vi "ZVisualize.vi"() -> ()   [LabVIEW 2016]
uses:
  <vilib>/Utility/miscctls.llb/LVPointDoubleTypeDef.ctl
  subVI/ZDataVIS_StateWire.ctl
  <vilib>/MakerHub/Toolbox/LMH-Toolbox.lvlib
  <userlib>/_OpenG.lib/array/array.llb/Reverse 2D Array (DBL)__ogtk.vi
panel:
  out "mem after unflatten":dbl
  out "mem before unflatten":dbl
  out "mem after load dat":dbl
  out "mem before load dat":dbl
  out "after 'graph smoething'":dbl
  out "before 'graph something'":dbl
  out "Vfast":dbl[](graph)
  in  "scannn names":string[](array[string])
  in  "IV setup":T1={"# of Vslow"=1, "# Vfast"=41, "#IV Curves at each gate"=1, "B/T offset"=0, "Discard first # curves"=0, "Manual offset"=0, "Field Period"=1, "# of fields/Temperatures"=1}
  in  "Vsd":u16(ring)=17 items=["time", "temp", "B", "Vsource", "Lockin0", "Lockin1", "Lockin2", "Lockin3", "Lockin4", "Lockin5", "B_rate", "DC0", "DC1", "DC2", "DC3", "DC4", "DC5", "DC6", "DC7", "LOCKIN INFO"]
  in  "I":u16(ring)=5 items=["time", "temp", "B", "Vsource", "Lockin0", "Lockin1", "Lockin2", "Lockin3", "Lockin4", "Lockin5", "B_rate", "DC0", "DC1", "DC2", "DC3", "DC4", "DC5", "DC6", "DC7", "LOCKIN INFO"]
  out "wiring":string[][](array[string])
  in  "loading":bool=TRUE
  in  "Tab Control":T2(tab)
  in  "Z Axis":T3(ring)=enum."dI/dV 2T"
  in  "Y AXIS":i32(listbox)=7
  in  "X AXIS":i32(listbox)=1
  in  "tpose":bool
  in  "-Z":bool
  in  "-X":bool
  in  "-Y":bool
  in  "-X rows or columns":enum16{"rows", "columns"}(ring)
  in  "color scale":u32[](array[colorbox])=[16711680, 16772608, 6618880, 3381759, 16860, 10420479]
  in  "autoName axes":bool=TRUE
  in  "auto chop IV":bool=TRUE
  in  "e^2/h?":bool
  in  "Filter data?":bool
  in  "Differential Bin":dbl=10.0
  in  "Fake Point Val":dbl format="%#_13g"
  in  "X Scale Selection":enum32{"Manual", "Auto"}(tab)=enum."Auto"
  in  "Manual CTLs":T4={"X Low"=-0.2, "X High"=0.2, "X Step Size"=0.0005} {"X Step Size" format="%#_6p"; "X High" format="%#_6p"; "X Low" format="%#_6p"}
  in  "Auto CTLs":cluster{"METHOD":bool, "Steps":dbl}={"METHOD"=FALSE, "Steps"=1000.0}
  in  "Sweep Cursor":bool
  out "y direction":i32=1000
  out "x direction":i32=41
  in  "x or y sweep":enum32{"X", "Y"}(radio)
  in  "ms to wait":u32=5
  in  "loop ctl":bool
  in  "GENERATE BEFORE VISUALIZING":bool=TRUE
  in  "DAT GENERATION PARAMETERS":T5(tab)
  in  "File Information":T6={"File or folder path (input)"=path "G:/My Drive/ansom/Data/PPMS2/SA03008L.20190612/004_SG_IV_Testing", "output file description"="test123"}
  in  "increment (T) or overwrite (F) folders":bool
  in  "offset":i32
  in  "length":i32=100000
  in  "Portion of data":cluster{dbl, dbl}(slide)={1.0, 0.0} scale=0.0..1.0
  in  "attempt to fix filtered time?":bool
  in  "decimating factor for generation":i32=1
  out "Source-drain Current vs Voltage":cluster{"Vfast":dbl[], dbl[]}(graph) caption="XY Graph"
  out "Source-drain Current vs Side Gate Voltage":cluster{"Vfast":dbl[], dbl[]}(graph) caption="XY Graph"
  in  "update":bool
  out "Field":dbl=-5.021235521235521
  out "slowest":dbl=0.20001035419657615
  out "2term Intensity":dbl[][](graph)
  in  "side points 4T":i32=8
  in  "side points 2T":i32=12
  in  "Field/Temperature":i32(slide) min=0 max=36 step=1 scale=-1.1..-1.0
  out "Data Selection":cluster{dbl[], dbl[]}(graph)
  in  "OK":bool
  in  "USELESS CONTROLS":u32(colorbox)=6618880
  # "<- necessary if trying to nab"
  # "for 7/18/18"
  # "The Wayside™"
  # "for 6/__/19"
  # "**These switches don't\nupdate the axes yet"
  # "#TODO: add reverse feature"
  # "For old data -v"
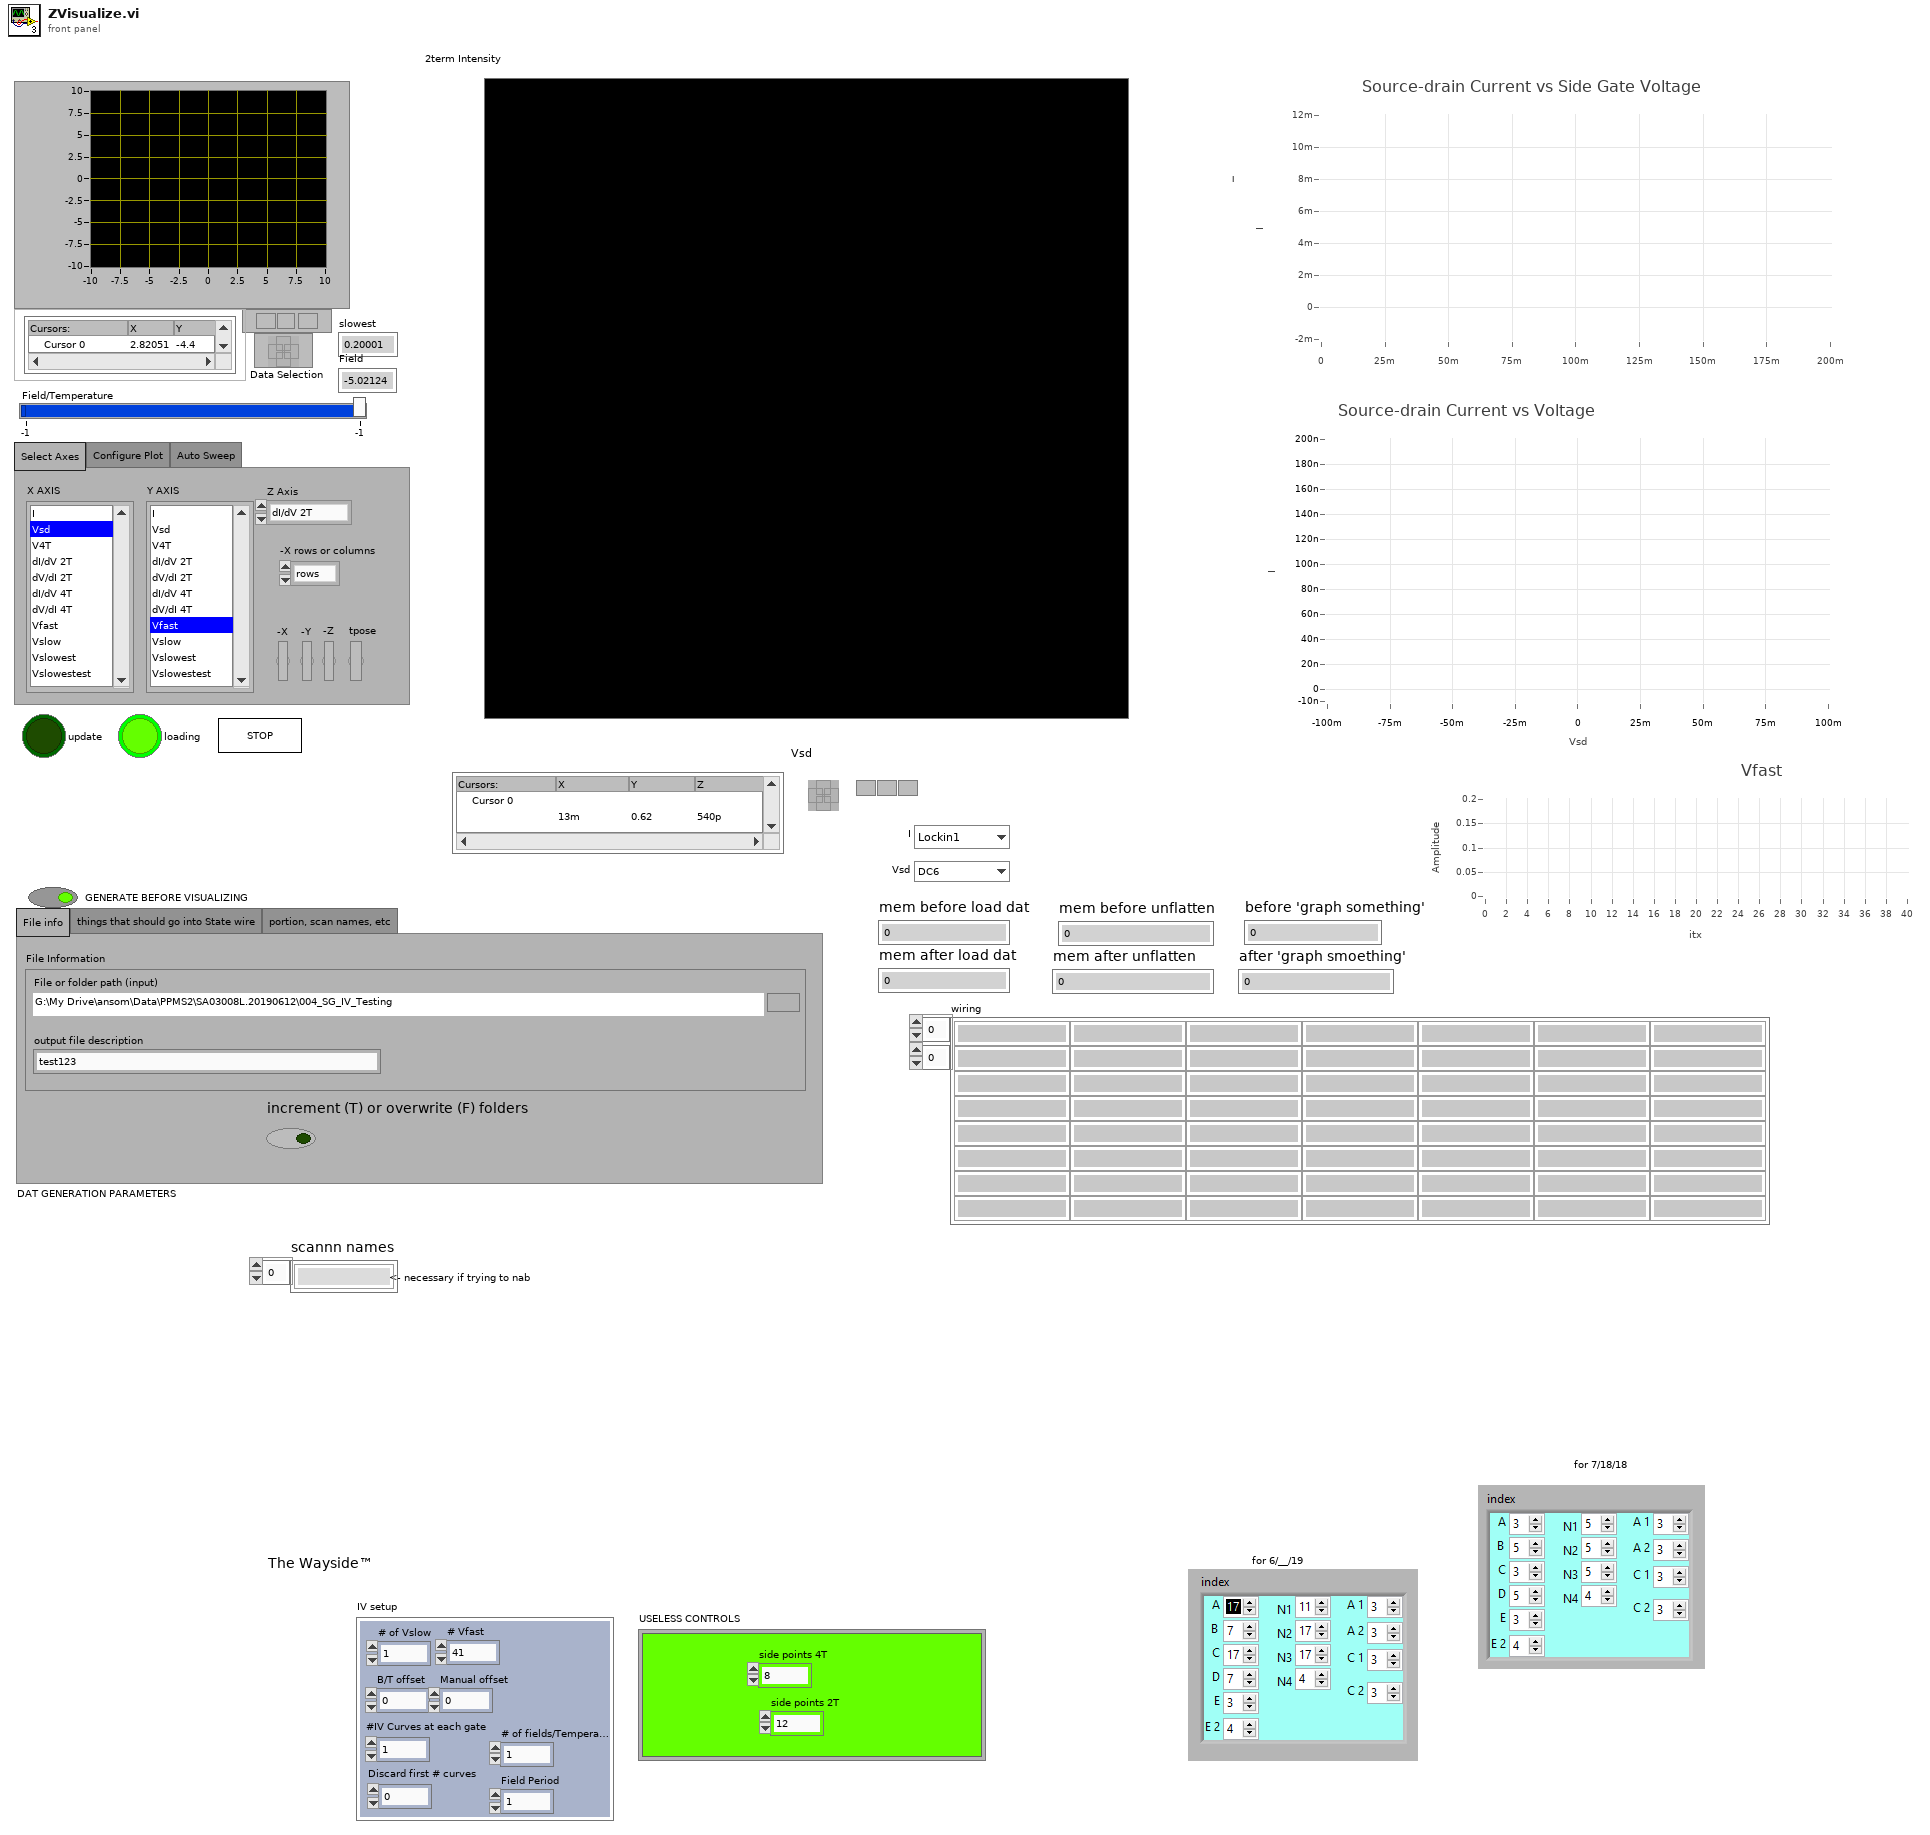
[diagram p1: front panel]
types:
  T1 = cluster{"# of Vslow":i32, "# Vfast":i32, "#IV Curves at each gate":i32, "B/T offset":i32, "Discard first # curves":i32, "Manual offset":i32, "Field Period":i32, "# of fields/Temperatures":i32}
  T2 = enum32{"Select Axes", "Configure Plot", "Auto Sweep"}
  T3 = enum16{"I", "Vsd", "V4T", "dI/dV 2T", "dV/dI 2T", "dV/dI 4T", "dI/dV 4T"}
  T4 = cluster{"X Low":dbl, "X High":dbl, "X Step Size":dbl}
  T5 = enum32{"File info", "things that should go into State wire", "portion, scan names, etc"}
  T6 = cluster{"File or folder path (input)":path, "output file description":string}
  T7 = enum32{"invalid app kind", "Development System", "Run Time System", "Student Edition", "Embedded LabVIEW", "Evaluation", "Custom"}
  T8 = cluster{"I":dbl[], "Vsd":dbl[], "V4T":dbl[], "dI/dV 2T":dbl[], "dV/dI 2T":dbl[], "dV/dI 4T":dbl[], "dI/dV 4T":dbl[]}[][][]
  T9 = enum32{"Invalid", "Standard", "Closed", "Hidden", "Minimized", "Maximized"}
  T10 = cluster{"# Vslow":i32, "# Vfast":i32, "# Vslowest":i32, "# Samples per IV":i32}
  T11 = typedef "ZDataVIS_StateWire.ctl" = cluster{"Core":cluster{"Current VI Reference":refnum<vi>, "Close Panel on Exit?":bool}, "Sweep Data Cluster":cluster{"Vfast":dbl[][], "Vslow":dbl[], "Vslowest":dbl[], "Comments":string, "Scan names":string[]}, "Cursor Info":cluster{"Fast Index":dbl[], "Slow Index":dbl, "Slow Indices":dbl[], "Raw Cursor Position":T12, "Field / temp":i32}, "Scan names":string[], "Data DVR":refnum<data-value>, "Arr of Y arrays (intensity info)":dbl[][], "Decimated X values":dbl[], "X Step Info":cluster{"X Low":dbl, "X High":dbl, "X Step":dbl}, "Voffset -2T":dbl, "Wiring Configuration ":string[][]}
  T12 = typedef "LVPointDoubleTypeDef.ctl" = cluster{"X":dbl, "Y":dbl}
  T13 = cluster{"Fast Index (Cursor X)":dbl[], "Slow Index (Cursor Y)":dbl, "Slow Indices":dbl[], "Raw Cursor Position":T12}
  T14 = cluster{"Vfast":dbl[][], "Vslow":dbl[], "Vslowest":dbl[], "Comments":string, "Scan names":string[]}
  T15 = cluster{"Current VI Reference":refnum<vi>, "Close Panel on Exit?":bool}
  T16 = typedef "Dictionary Object RefNum__ogtk.ctl" = refnum<k1>
  T17 = cluster{"IV":cluster{dbl[], dbl[]}[][][], "IV-2T":cluster{dbl[], dbl[]}[][][], "Vfast":dbl[][], "Vslow":dbl[], "Vslowest":dbl[], "Comments":string, "Scan names":string[]}[]
  T18 = cluster{"IV":cluster{dbl[], dbl[]}[][][], "IV-2T":cluster{dbl[], dbl[]}[][][], "Vfast":dbl[][], "Vslow":dbl[], "Vslowest":dbl[], "Comments":string, "Scan names":string[]}
  T19 = cluster{"Value":i32, "Value":i32, "Value":enum16{"I", "Vsd", "V4T", "dI/dV 2T", "dV/dI 2T", "dV/dI 4T", "dI/dV 4T"}}
  T20 = cluster{"Slow Index":dbl, "Field/Temperature":i32, dbl}
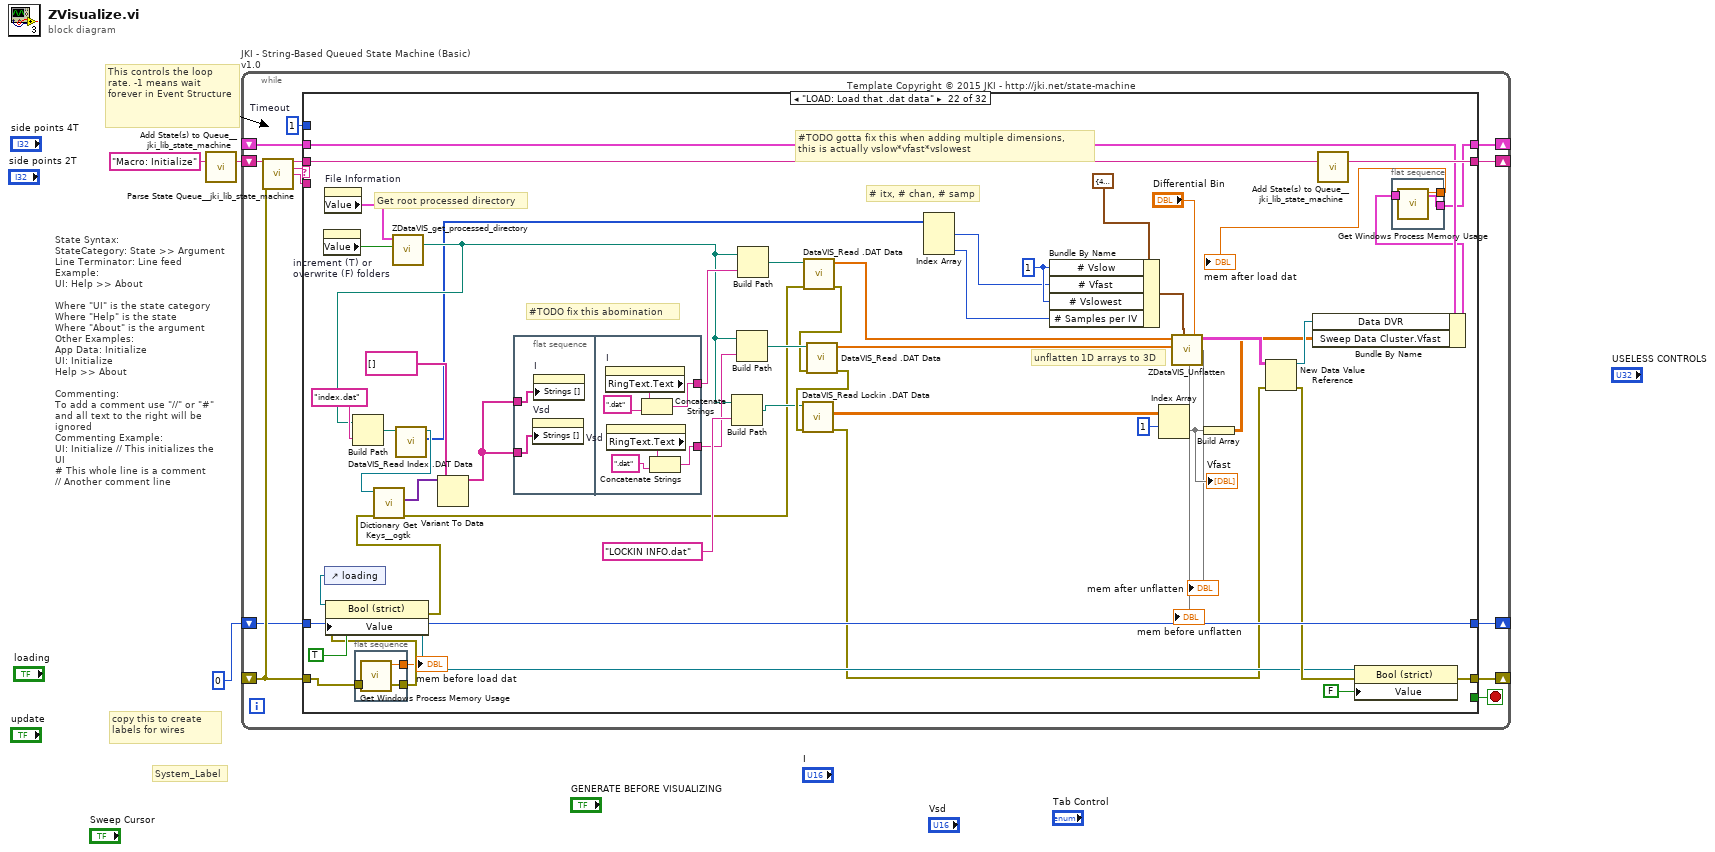
[diagram p0: block diagram]
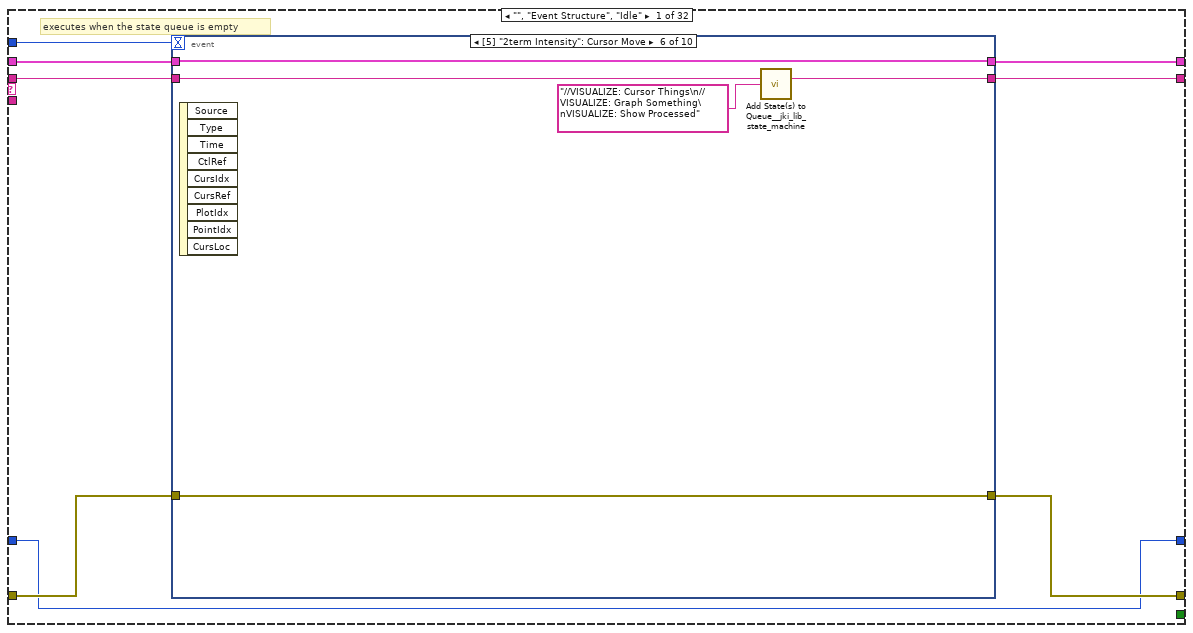
[diagram p2: hidden frame]
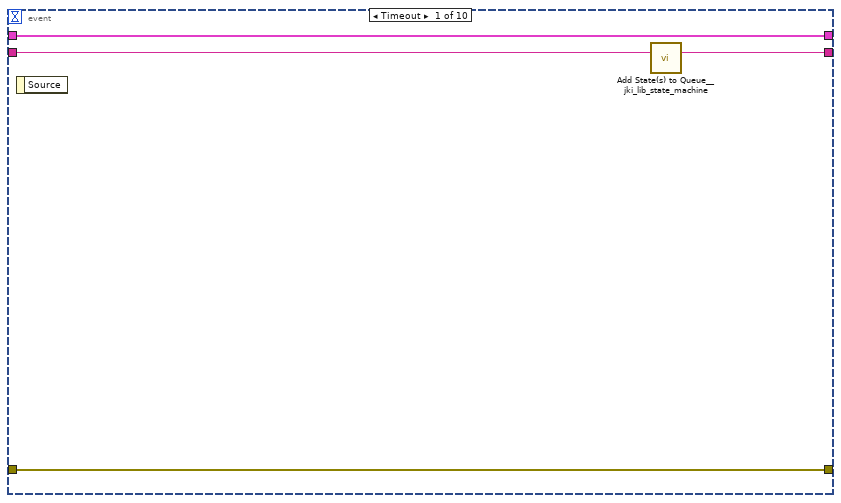
[diagram p3: hidden frame]
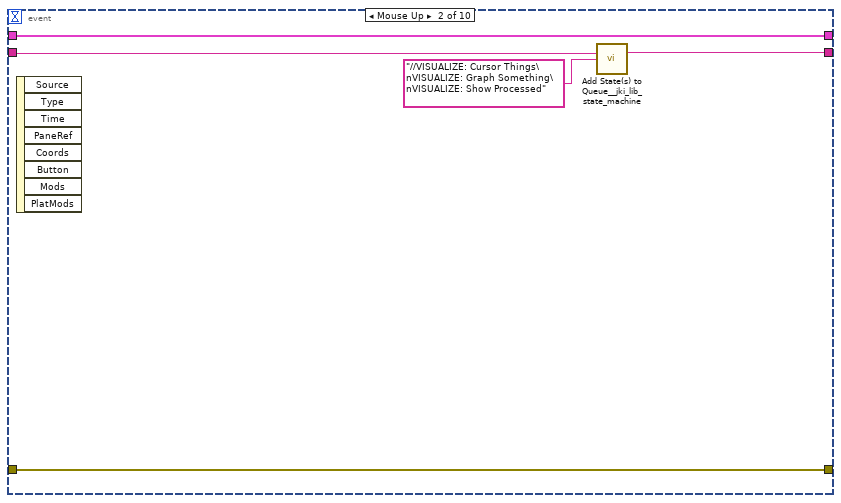
[diagram p4: hidden frame]
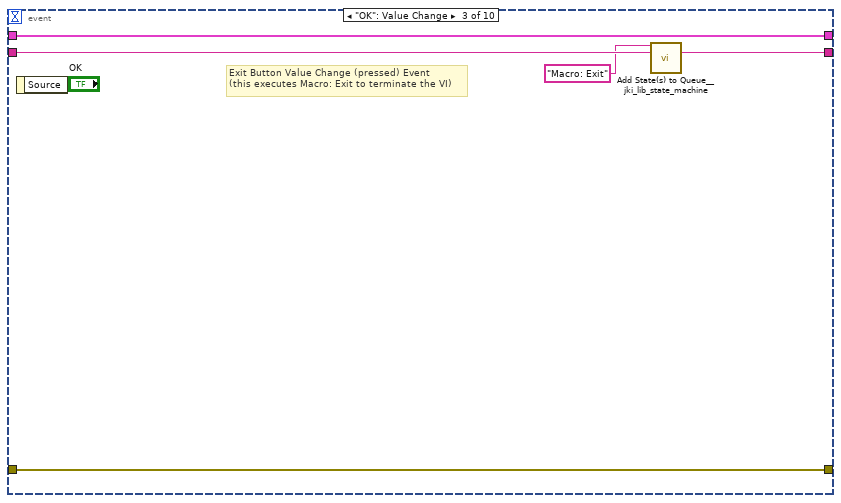
[diagram p5: hidden frame]
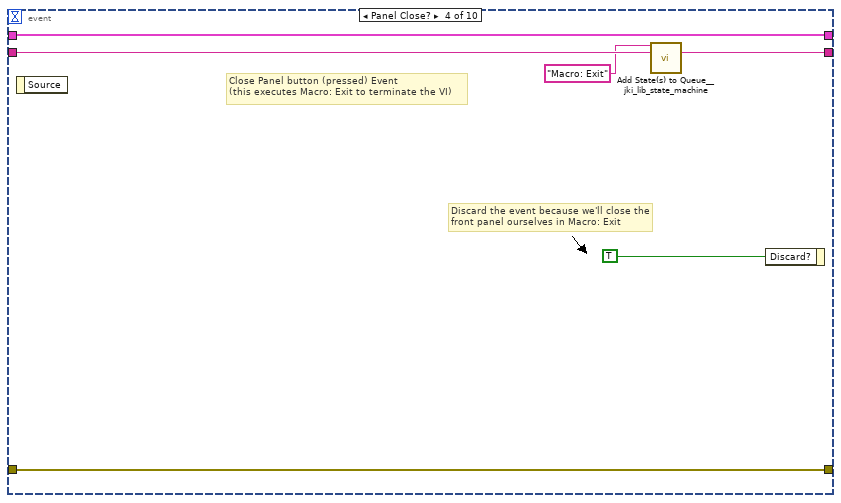
[diagram p6: hidden frame]
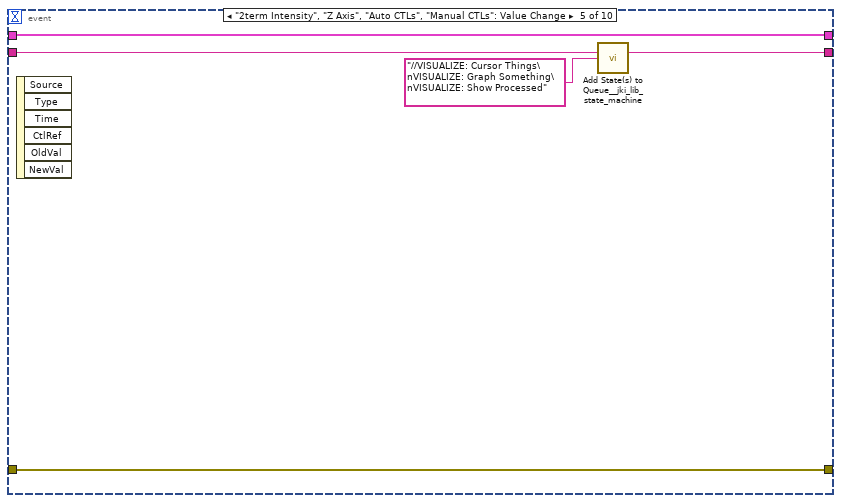
[diagram p7: hidden frame]
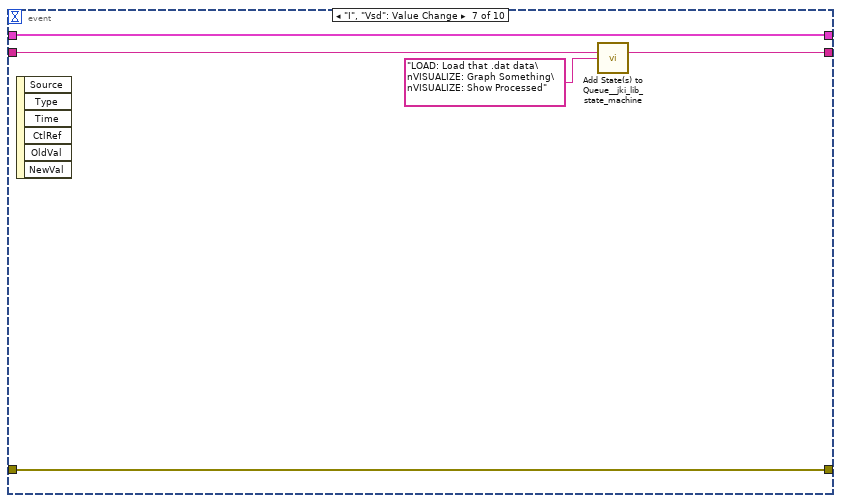
[diagram p8: hidden frame]
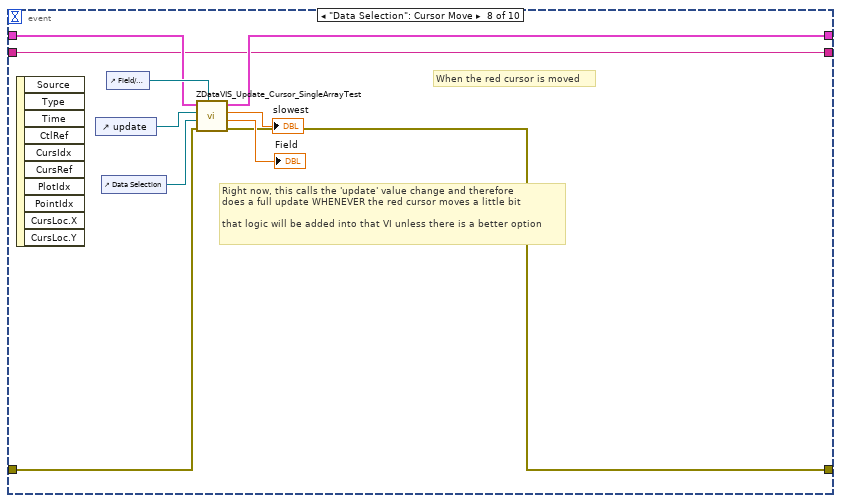
[diagram p9: hidden frame]
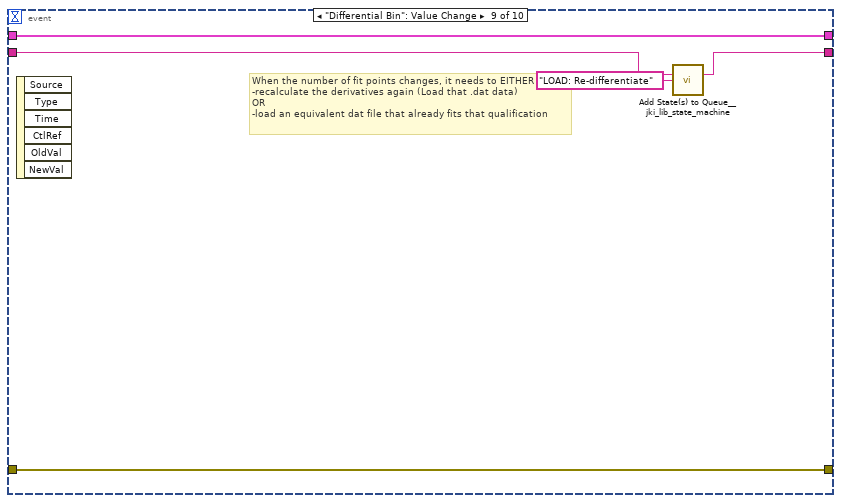
[diagram p10: hidden frame]
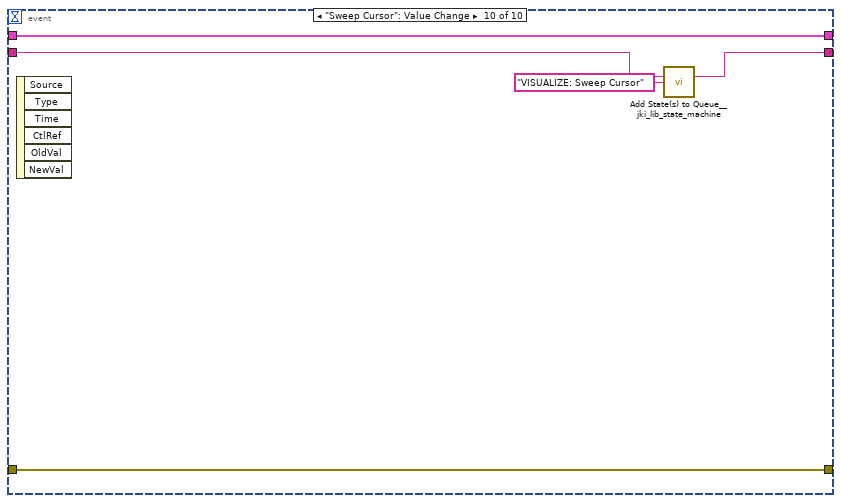
[diagram p11: hidden frame]
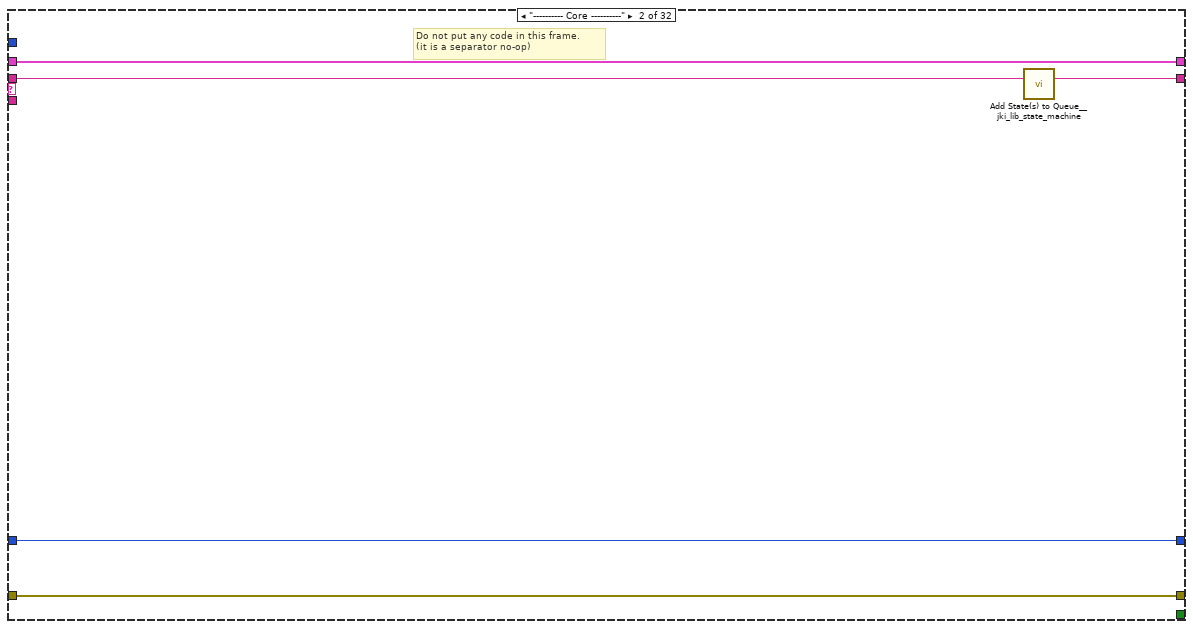
[diagram p12: hidden frame]
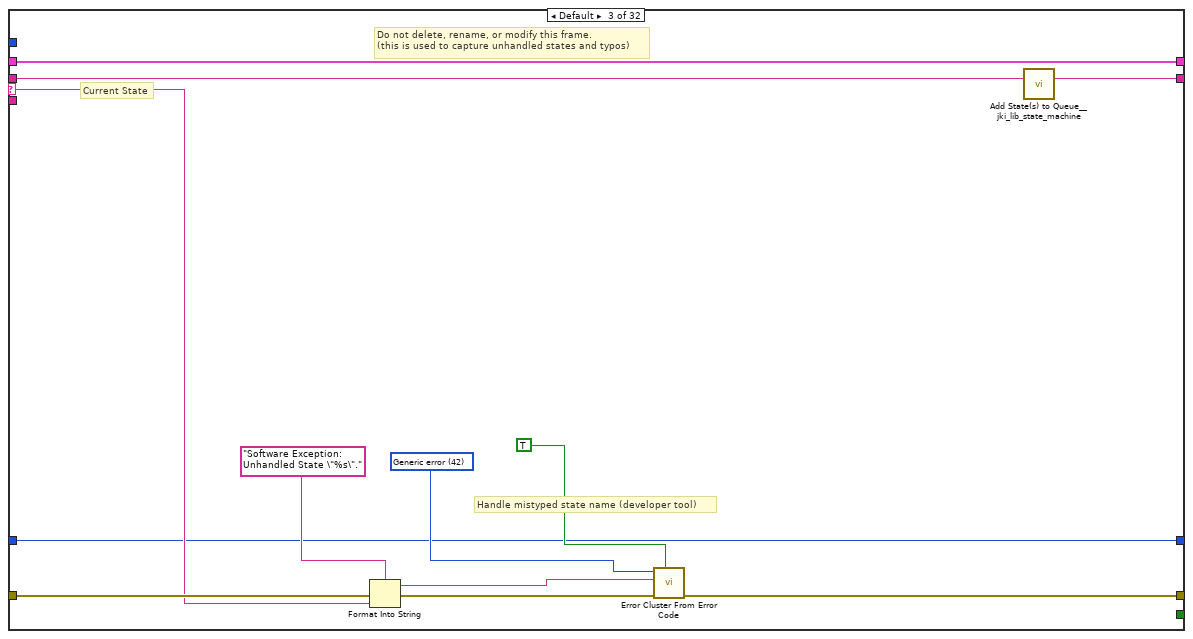
[diagram p13: hidden frame]
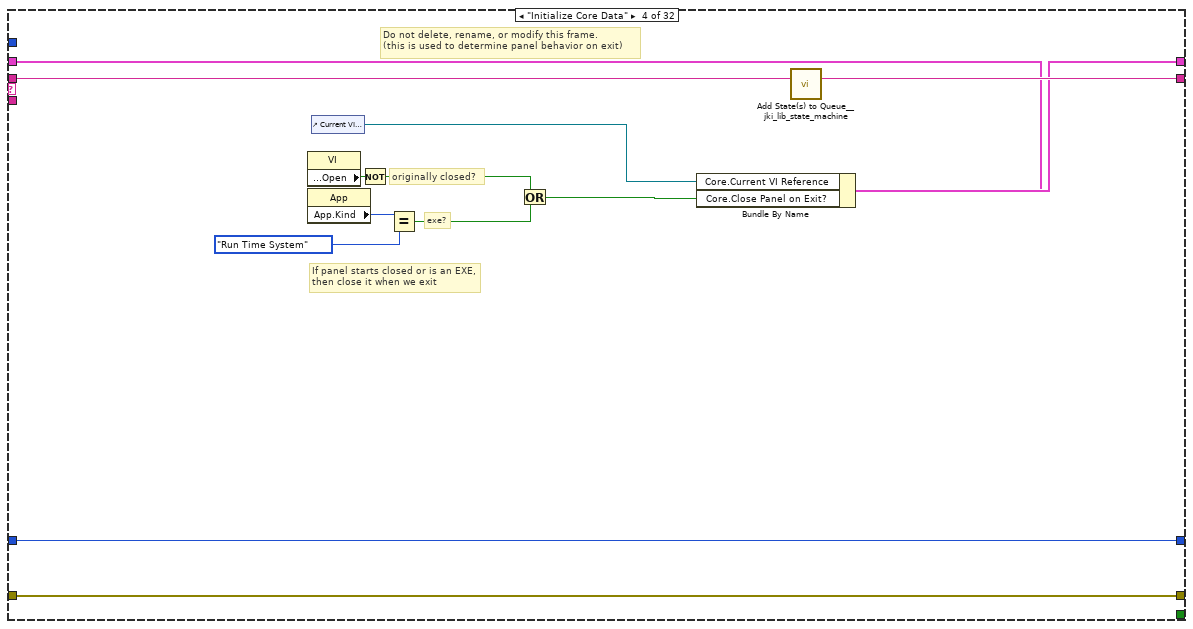
[diagram p14: hidden frame]
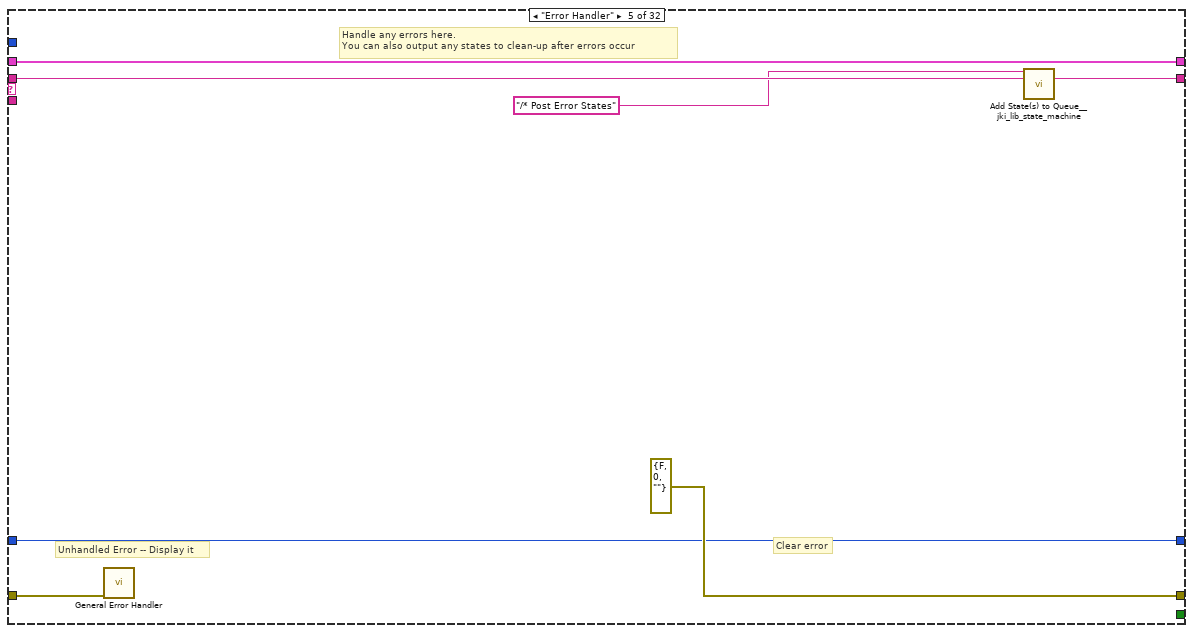
[diagram p15: hidden frame]
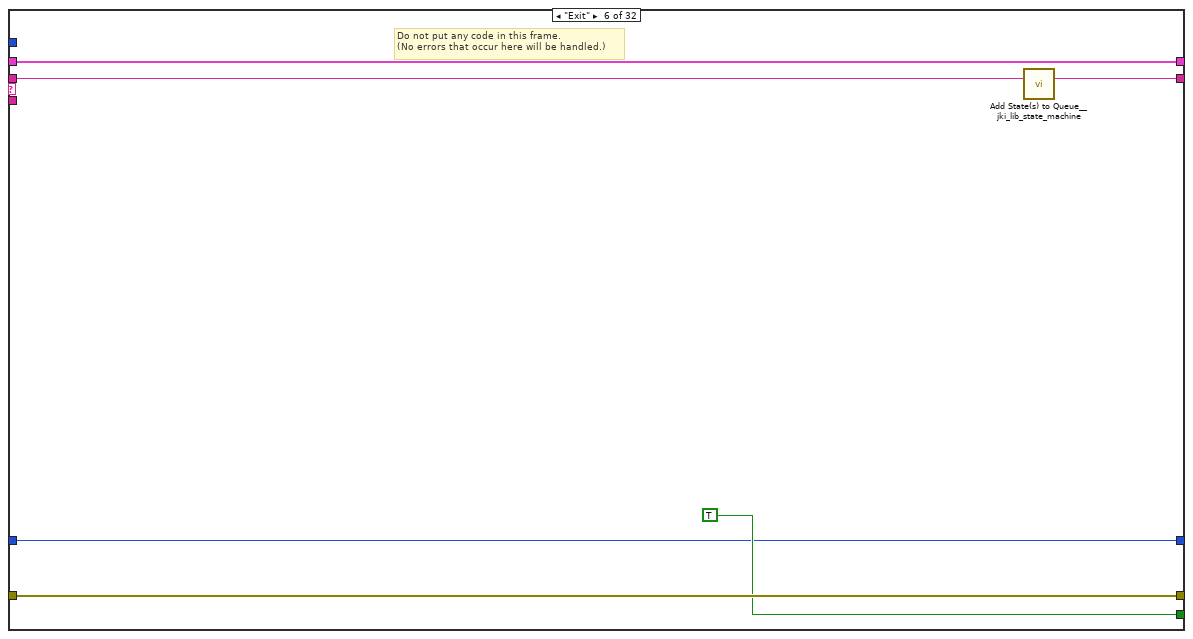
[diagram p16: hidden frame]
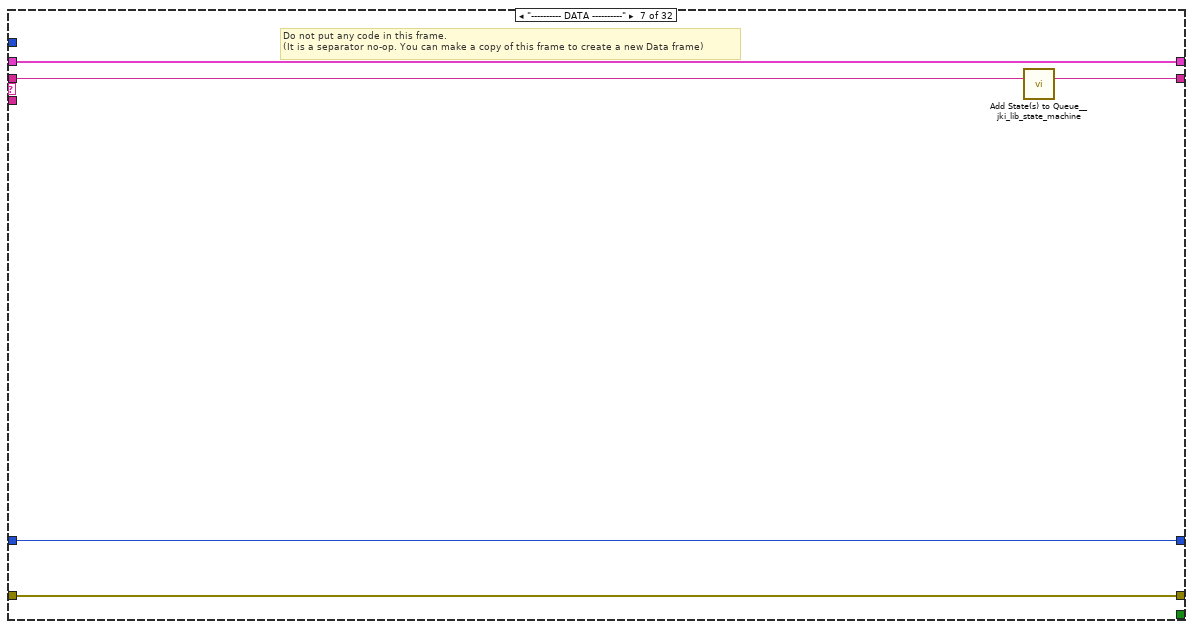
[diagram p17: hidden frame]
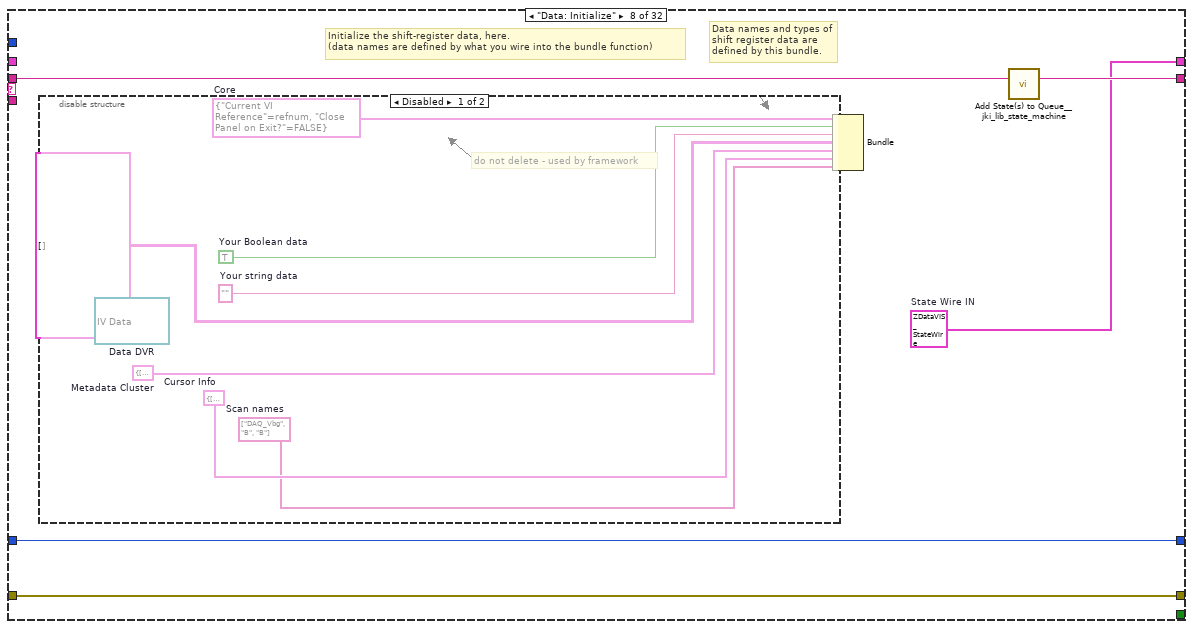
[diagram p18: hidden frame]
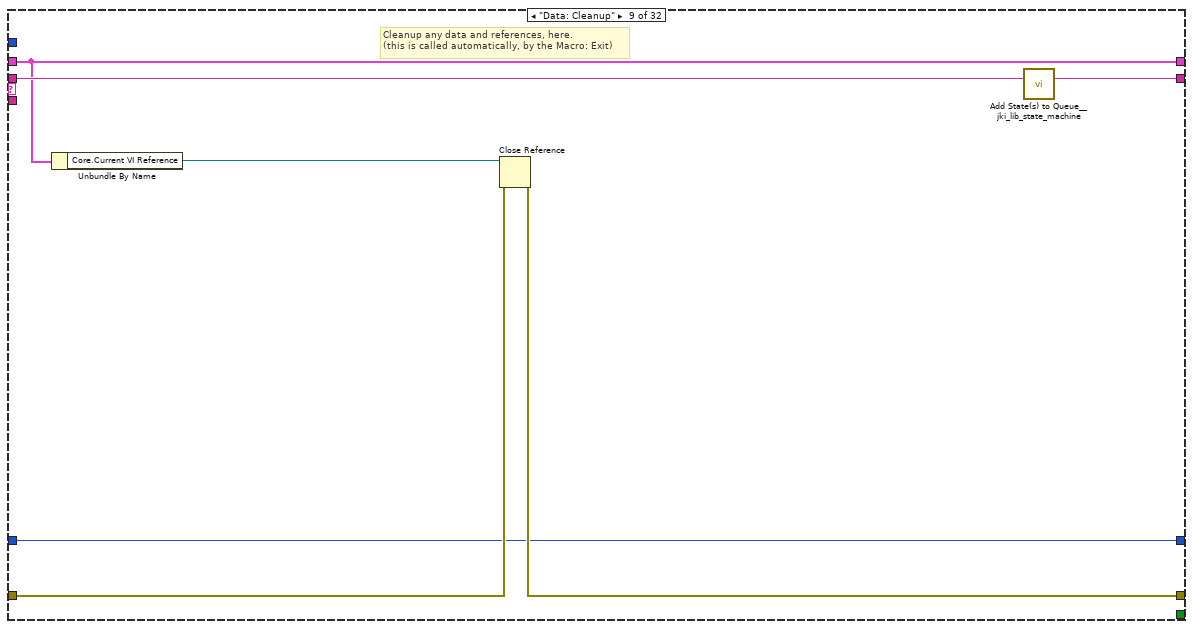
[diagram p20: hidden frame]
diagram:
  # "State Syntax:\nStateCategory: State >> Argument\nLine Terminator: Line feed\nExample:\nUI: Help >> About\n\nWhere \"UI\" is the state category\nWhere \"Help\" is the state\nWhere \"About\" is the argument\nOther Examples:\nApp Data: Initialize\nUI: Initialize\nHelp >> About\n\nCommenting:\nTo add a comment use \"//\" or \"#\" and all text to the right will be ignored\nCommenting Example:\nUI: Initialize // This initializes the UI\n# This whole line is a comment\n// Another comment line"
  # "copy this to create labels for wires"
  # "This controls the loop rate. -1 means wait forever in Event Structure"
  # "System_Label"
  n1 = call <vilib>:"Add State(s) to Queue__jki_lib_state_machine.vi"("State(s) in (\"\")"="Macro: Initialize") -> ("States Out"=w3:string)  [unwired: 14 in]
  n2 = while "JKI - String-Based Queued State Machine (Basic) v1.0" {
    shift-right: [w9] -> _
    shift-left: _ -> [w8]
    shift-right: [w12] -> _
    shift-left: _ -> [w6]
    shift-right: [w11] -> _
    shift-left: w3 -> [w13]
    shift-right: [w4] -> _
    shift-left: 0 -> [w5]
    stop <- w10 stop-if-true
    w7 = 1  # Timeout
    # "Template Copyright © 2015 JKI - http://jki.net/state-machine"
    n3 = call <vilib>:"Parse State Queue__jki_lib_state_machine.vi"("State Queue"=w13, "Error In (no error)"=w6) -> ("Remaining States"=w15:string, "Current State"=w16:string, "Arguments"=w14:string)  [unwired: 11 in]
    n4 = case shown="\"LOAD: Load that .dat data\"" w16 {
      selector: w16 -> [_ _ w86 _ _ _ _ _ _ _ _ _ _ _ _ _ _ _ _ _ _ _ _ _ _ _ _ _ _ _ _ _]
      tunnel: w15 -> [w24 w84 w90 w109 w116 w122 w127 w132 w146 w151 w156 w163 w175 w202 w208 w219 w231 w243 w248 w260 w265 w318 w358 w366 w396 w407 w434 w485 w499 w560 w568 w589]
      tunnel: w14 -> [_ _ _ _ _ _ _ _ _ _ _ w158 w169 _ _ _ _ _ _ _ _ _ _ _ _ _ _ _ _ _ _ _]
      tunnel: w8 -> [w22 w81 w88 w100 w113 w120 w124 _ w141 w148 w154 w161 w171 w199 w205 w216 w229 w240 w245 w258 w263 w316 w354 w362 w393 w404 w432 w469 w500 w557 w565 w587]
      tunnel: [w21 w82 w92 w106 errorcluster {"status"=FALSE, "code"=0, "source"=""} ("error out") w119 w125 w130 w142 w149 w153 w159 w172 w200 w206 w217 w226 w241 w246 w249 w262 w313 w336 w361 w385 w405 w417 w471 w501 w558 w566 w576] -> w12
      tunnel: w6 -> [w20 w82 w91 w106 w112 w119 w125 w130 w143 w149 w153 w160 w173 w200 w206 w217 w225 w241 w246 w256 w262 w273 w339 w361 w388 w405 w416 w472 w502 w558 w566 w577]
      tunnel: [w23 w83 w89 w108 w115 w121 w126 w131 w145 w150 w155 w162 w174 w201 w207 w218 w230 w242 w247 w259 w264 w317 w357 w365 w395 w406 w433 w484 w498 w559 w567 w588] -> w11
      tunnel: [_ _ _ _ _ TRUE _ _ _ _ _ _ _ _ _ _ _ _ _ _ _ _ _ _ _ _ _ _ _ _ _ _] -> w10
      tunnel: [w19 w81 w88 w107 w113 w120 w124 w129 w141 w148 w154 w161 w171 w199 w205 w216 w229 w240 w245 w258 w263 w269 w353 w364 w392 w404 w432 w468 w495 w557 w565 w587] -> w9
      tunnel: w7 -> [w18 _ _ _ _ _ _ _ _ _ _ _ _ _ _ _ _ _ _ _ _ _ _ _ _ _ _ _ _ _ _ _]
      tunnel: w5 -> [w17 w80 w85 w97 w110 w117 w123 w128 w140 w147 w152 w157 w168 w198 w203 w209 w228 w232 w244 w257 w261 w315 w340 w363 w390 w403 w423 w467 w493 w556 w561 w570]
      tunnel: [w17 w80 w85 w97 w110 w117 w123 w128 w140 w147 w152 w157 w168 w198 w203 w209 w228 w232 w244 w257 w261 w315 w340 w363 w390 w403 w426 w467 w493 w556 w561 w570] -> w4
      frame "", "Event Structure", "Idle" {
        # "executes when the state queue is empty"
        n5 = event shown="[5] \"2term Intensity\": Cursor Move" {
          selector: _ -> [_ _ _ _ _ _ _ _ _ _]
          dyn-events: _ -> [_ _ _ _ _ _ _ _ _ _]
          timeout: w18 -> [_ _ _ _ _ _ _ _ _ _]
          tunnel: w24 -> [w28 w32 w38 w44 w47 w52 w57 w64 w72 w76]
          tunnel: [w27 w30 w37 w43 w45 w50 w55 w64 w71 w75] -> w23
          tunnel: w22 -> [w25 w31 w35 w41 w49 w54 w59 w66 w73 w78]
          tunnel: [w26 w29 w36 w42 w48 w53 w58 w61 w74 w79] -> w21
          tunnel: w20 -> [w26 w29 w36 w42 w48 w53 w58 w63 w74 w79]
          tunnel: [w25 w31 w35 w41 w49 w54 w59 w65 w73 w78] -> w19
          event Timeout {
            n6 = event-data() -> ()  [unwired: 1 in, 1 out]
            n7 = call <vilib>:"Add State(s) to Queue__jki_lib_state_machine.vi"("State(s) in (\"\")"=w28) -> ("States Out"=w27:string)  [unwired: 14 in]
          }
          event Mouse Up {
            n8 = event-data() -> ()  [unwired: 1 in, 8 out]
            n9 = call <vilib>:"Add State(s) to Queue__jki_lib_state_machine.vi"("State(s) in (\"\")"=w32, "State(s) at Back (\"\")"="//VISUALIZE: Cursor Things\nVISUALIZE: Graph Something\nVISUALIZE: Show Processed" ("State(s) at Back (\"\")")) -> ("States Out"=w30:string)  [unwired: 13 in]
          }
          event "OK": Value Change {
            # "Exit Button Value Change (pressed) Event\n(this executes Macro: Exit to terminate the VI)"
            n10 = event-data() -> ()  [unwired: 1 in, 1 out]
            n11 = call <vilib>:"Add State(s) to Queue__jki_lib_state_machine.vi"("State(s) in Front (\"\")"="Macro: Exit", "State(s) in (\"\")"=w38) -> ("States Out"=w37:string)  [unwired: 13 in]
          }
          event Panel Close? {
            # "Discard the event because we'll close the front panel ourselves in Macro: Exit"
            # "Close Panel button (pressed) Event\n(this executes Macro: Exit to terminate the VI)"
            n12 = event-data() -> ()  [unwired: 1 in, 1 out]
            n13 = call <vilib>:"Add State(s) to Queue__jki_lib_state_machine.vi"("State(s) in Front (\"\")"="Macro: Exit", "State(s) in (\"\")"=w44) -> ("States Out"=w43:string)  [unwired: 13 in]
            n14 = event-data("Discard?"=TRUE) -> ()  [unwired: 1 in, 1 out]
          }
          event "2term Intensity", "Z Axis", "Auto CTLs", "Manual CTLs": Value Change {
            n15 = event-data() -> ()  [unwired: 1 in, 6 out]
            n16 = call <vilib>:"Add State(s) to Queue__jki_lib_state_machine.vi"("State(s) in (\"\")"=w47, "State(s) at Back (\"\")"="//VISUALIZE: Cursor Things\nVISUALIZE: Graph Something\nVISUALIZE: Show Processed" ("State(s) at Back (\"\")")) -> ("States Out"=w45:string)  [unwired: 13 in]
          }
          event "2term Intensity": Cursor Move {
            n17 = event-data() -> ()  [unwired: 1 in, 9 out]
            n18 = call <vilib>:"Add State(s) to Queue__jki_lib_state_machine.vi"("State(s) in (\"\")"=w52, "State(s) at Back (\"\")"="//VISUALIZE: Cursor Things\n//VISUALIZE: Graph Something\nVISUALIZE: Show Processed" ("State(s) at Back (\"\")")) -> ("States Out"=w50:string)  [unwired: 13 in]
          }
          event "I", "Vsd": Value Change {
            n19 = event-data() -> ()  [unwired: 1 in, 6 out]
            n20 = call <vilib>:"Add State(s) to Queue__jki_lib_state_machine.vi"("State(s) in (\"\")"=w57, "State(s) at Back (\"\")"="LOAD: Load that .dat data\nVISUALIZE: Graph Something\nVISUALIZE: Show Processed" ("State(s) at Back (\"\")")) -> ("States Out"=w55:string)  [unwired: 13 in]
          }
          event "Data Selection": Cursor Move {
            # "Right now, this calls the 'update' value change and therefore \ndoes a full update WHENEVER the red cursor moves a little bit\n\nthat logic will be added into that VI unless there is a better option"
            # "When the red cursor is moved"
            n21 = event-data() -> ()  [unwired: 1 in, 10 out]
            n22 = control-ref of="update"() -> (w62:refnum<vi>)
            n23 = control-ref of="Data Selection"() -> (w68:refnum<vi>)
            n24 = control-ref of="Field/Temperature"() -> (w67:refnum<vi>)
            n25 = call "ZDataVIS_Update_Cursor_SingleArrayTest.vi"("Field/Temperature 2"=w67, "error in (no error)"=w63, "Cursor Graph"=w68, "update bool"=w62, "State Wire IN 2"=w66) -> ("error out"=w61:errorcluster, "Field"=→"Field":dbl, "slowest"=→"slowest":dbl, "State Wire IN 3"=w65:T11)  [unwired: 3 in]
          }
          event "Differential Bin": Value Change {
            # "When the number of fit points changes, it needs to EITHER\n-recalculate the derivatives again (Load that .dat data)\nOR\n-load an equivalent dat file that already fits that qualification"
            n26 = event-data() -> ()  [unwired: 1 in, 6 out]
            n27 = call <vilib>:"Add State(s) to Queue__jki_lib_state_machine.vi"("State(s) in (\"\")"=w72, "State(s) at Back (\"\")"="LOAD: Re-differentiate" ("State(s) at Back (\"\")")) -> ("States Out"=w71:string)  [unwired: 13 in]
          }
          event "Sweep Cursor": Value Change {
            n28 = event-data() -> ()  [unwired: 1 in, 6 out]
            n29 = call <vilib>:"Add State(s) to Queue__jki_lib_state_machine.vi"("State(s) in (\"\")"=w76, "State(s) at Back (\"\")"="VISUALIZE: Sweep Cursor" ("State(s) at Back (\"\")")) -> ("States Out"=w75:string)  [unwired: 13 in]
          }
        }
      }
      frame "---------- Core ----------" {
        # "Do not put any code in this frame.\n(it is a separator no-op)"
        n30 = call <vilib>:"Add State(s) to Queue__jki_lib_state_machine.vi"("State(s) in (\"\")"=w84) -> ("States Out"=w83:string)  [unwired: 14 in]
      }
      frame Default {
        w95 = 42 items=["No error", "Argument error", "Memory is full", "Out of zone", "End of file", "File already open", "Generic file I/O error", "File not found", "File permission error", "Disk is full", "Duplicate path", "Too many files open", "System feature not enabled", "Resource file not found", "Cannot add resource", "Resource not found", "Image not found", "Image memory error", "Pen does not exist", "Config type invalid", "Config token not found", "Config parse error", "Config memory error", "Bad external code format", "Bad external code offset", "External code not present", "Null window", "Destroy window error", "Null menu", "Print aborted", "Bad print record", "Print driver error", "Windows error during printing", "Memory error during printing", "Print dialog error", "Generic print error", "Invalid device refnum", "Device not found", "Device parameter error", "Device unit error", "Cannot open device", "Device call aborted", "Generic error", "Cancelled by user", "Object ID too low", "Object ID too high", "Object not in heap", "Unknown heap", "Unknown object (invalid DefProc)", "Unknown object (DefProc not in table)", "Message out of range", "Invalid (null) method", "Unknown message", "Manager call not supported", "Bad address", "Network operation in progress", "Network operation timed out", "Connection is busy", "Network attribute not supported", "Network error", "Address in use", "System out of memory", "Connection aborted", "Connection refused", "Not connected", "Already connected", "Connection closed", "Initialization error (interapplication manager)", "Bad occurrence", "Wait on unbound occurrence handler", "Occurrence queue overflow", "Datalog type conflict", "Unused", "Unrecognized type (interapplication manager)", "Memory corrupt", "Failed to make temporary DLL", "Old CIN version", "Drag socket not found", "Failed to load drop-object", "Failed to register OLE object", "Failed to release OLE object", "Format specifier type mismatch", "Unknown format specifier", "Too few format specifiers", "Too many format specifiers", "Scan failed", "Newer CIN version", "Error converting to variant", "Runtime menu error", "Password tampered", "Variant attribute not found", "Incompatible variant data type", "Event data is not available", "Event Store is not present", "Occurrence is not found", "Event Queue is not created", "Event info is not available", "Refnum passed is NULL", "Error retrieving Class GUID", "Error retrieving CoClass GUID", "Error retrieving TypeLib GUID.", "Bad built application magic bytes.", "Specific driver is different from the specific driver associated with the Logical Name.", "There is no session opened to the class driver.", "Max Error", "MAX - Error with config objects", "MAX - Error loading configuration", "MAX - Group not supported"]
        # "Current State"
        # "Do not delete, rename, or modify this frame.\n(this is used to capture unhandled states and typos)"
        # "Handle mistyped state name (developer tool)"
        n31 = Format Into String(format string="Software Exception: Unhandled State \"%s\"." ("message"), error in=w91, w86) -> (resulting string=w94:string, error out=w93:errorcluster)  [unwired: 1 in]
        n32 = call <vilib>:"Error Cluster From Error Code.vi"("show call chain? (False)"=TRUE, "error in (no error)"=w93, "error message (\"\")"=w94, "error code (0)"=w95) -> ("error out"=w92:errorcluster)  [unwired: 5 in]
        n33 = call <vilib>:"Add State(s) to Queue__jki_lib_state_machine.vi"("State(s) in (\"\")"=w90) -> ("States Out"=w89:string)  [unwired: 14 in]
      }
      frame "Initialize Core Data" {
        # "Do not delete, rename, or modify this frame.\n(this is used to determine panel behavior on exit)"
        # "originally closed?"
        # "exe?"
        # "If panel starts closed or is an EXE, then close it when we exit"
        n34 = property class="VI"() -> ("Front Panel.Open"=w105:bool)  [unwired: 2 in, 2 out]
        n35 = property class="App"() -> ("App.Kind"=w104:T7)  [unwired: 2 in, 2 out]
        n36 = control-ref of="Current VI Reference"() -> (w98:refnum<vi>)
        n37 = Not(x=w105) -> (.not. x?=w102:bool)
        n38 = Equal?(x=w104, y=T7."Run Time System" ("Application:Kind")) -> (x = y?=w101:bool)
        n39 = Or(x=w102, y=w101) -> (x .or. y?=w99:bool)
        n40 = Bundle By Name(cluster=w100, "Core.Current VI Reference"=w98, "Core.Close Panel on Exit?"=w99) -> (w107:T11)
        n41 = call <vilib>:"Add State(s) to Queue__jki_lib_state_machine.vi"("State(s) in (\"\")"=w109) -> ("States Out"=w108:string)  [unwired: 14 in]
      }
      frame "Error Handler" {
        # "Unhandled Error -- Display it"
        # "Handle any errors here.\nYou can also output any states to clean-up after errors occur"
        # "Clear error"
        n42 = call <vilib>:"General Error Handler.vi"("error in (no error)"=w112) -> ()  [unwired: 10 in, 5 out]
        n43 = call <vilib>:"Add State(s) to Queue__jki_lib_state_machine.vi"("State(s) in Front (\"\")"="/* Post Error States", "State(s) in (\"\")"=w116) -> ("States Out"=w115:string)  [unwired: 13 in]
      }
      frame "Exit" {
        # "Do not put any code in this frame.\n(No errors that occur here will be handled.)"
        n44 = call <vilib>:"Add State(s) to Queue__jki_lib_state_machine.vi"("State(s) in (\"\")"=w122) -> ("States Out"=w121:string)  [unwired: 14 in]
      }
      frame "---------- DATA ----------" {
        # "Do not put any code in this frame.\n(It is a separator no-op. You can make a copy of this frame to create a new Data frame)"
        n45 = call <vilib>:"Add State(s) to Queue__jki_lib_state_machine.vi"("State(s) in (\"\")"=w127) -> ("States Out"=w126:string)  [unwired: 14 in]
      }
      frame "Data: Initialize" {
        w129 = T11 {"Core"={"Current VI Reference"=refnum, "Close Panel on Exit?"=FALSE}, "Sweep Data Cluster"={"Vfast"=[], "Vslow"=[], "Vslowest"=[], "Comments"="", "Scan names"=[]}, "Cursor Info"={"Fast Index"=[], "Slow Index"=0.0, "Slow Indices"=[], "Raw Cursor Position"={"X"=0.0, "Y"=0.0}, "Field / temp"=0}, "Scan names"=[], "Data DVR"=refnum, "Arr of Y arrays (intensity info)"=[], "Decimated X values"=[], "X Step Info"={"X Low"=-0.1, "X High"=0.1, "X Step"=4e-05}, "Voffset -2T"=0.0, "Wiring Configuration "=[]}  # State Wire IN
        # "Data names and types of shift register data are defined by this bundle."
        # "Initialize the shift-register data, here.\n(data names are defined by what you wire into the bundle function)"
        n46 = disable-structure shown="Disabled" {
          frame Disabled {
            w134 = string[] ["DAQ_Vbg", "B", "B"]  # Scan names
            w135 = T13 {"Fast Index (Cursor X)"=[], "Slow Index (Cursor Y)"=0.0, "Slow Indices"=[], "Raw Cursor Position"={"X"=0.0, "Y"=0.0}}  # Cursor Info
            w136 = T14 {"Vfast"=[], "Vslow"=[], "Vslowest"=[], "Comments"="", "Scan names"=[]}  # Metadata Cluster
            (unwired) refnum<data-value> refnum  # Data DVR
            w137 = T15 {"Current VI Reference"=refnum, "Close Panel on Exit?"=FALSE}  # Core
            w138 = ""  # Your string data
            w139 = TRUE  # Your Boolean data
            # "do not delete - used by framework"
            n47 = Bundle("Core"=w137, "Your Boolean data"=w139, "Your string data"=w138, "Data Cell"=T8 [], "Metadata Cluster"=w136, "Cursor Info"=w135, "Scan names"=w134) -> ()  [unwired: 1 in, 1 out]
          }
          frame Enabled {
          }
        }
        n48 = call <vilib>:"Add State(s) to Queue__jki_lib_state_machine.vi"("State(s) in (\"\")"=w132) -> ("States Out"=w131:string)  [unwired: 14 in]
      }
      frame "Data: Cleanup" {
        # "Cleanup any data and references, here.\n(this is called automatically, by the Macro: Exit)"
        n49 = Unbundle By Name(w141) -> ("Core.Current VI Reference"=w144:refnum<vi>)
        n50 = Close Reference(reference=w144, error in (no error)=w143) -> (error out=w142:errorcluster)
        n51 = call <vilib>:"Add State(s) to Queue__jki_lib_state_machine.vi"("State(s) in (\"\")"=w146) -> ("States Out"=w145:string)  [unwired: 14 in]
      }
      frame "---------- UI ----------" {
        # "Do not put any code in this frame.\n(It is a separator no-op. You can make a copy of this frame to create a new UI frame)"
        n52 = call <vilib>:"Add State(s) to Queue__jki_lib_state_machine.vi"("State(s) in (\"\")"=w151) -> ("States Out"=w150:string)  [unwired: 14 in]
      }
      frame "UI: Initialize" {
        # "Initialize the User Interface, here.\n(this is called automatically, by the Macro: Init)"
        n53 = call <vilib>:"Add State(s) to Queue__jki_lib_state_machine.vi"("State(s) in (\"\")"=w156) -> ("States Out"=w155:string)  [unwired: 14 in]
      }
      frame "UI: Cursor Set" {
        # "Argument"
        # "Set and Unset Cursor Busy.\n(Usage: \"UI: Cursor Set >> Busy|Idle\")"
        n54 = case shown="\"Idle\", Default" w158 {
          tunnel: w160 -> [w165 w167]
          tunnel: [w164 w166] -> w159
          frame "Idle", Default {
            n55 = call <vilib>:"Unset Busy.vi"("error in (no error)"=w165) -> ("error out"=w164:errorcluster)  [unwired: 10 in]
          }
          frame "Busy" {
            n56 = call <vilib>:"Set Busy.vi"("error in (no error)"=w167) -> ("error out"=w166:errorcluster)  [unwired: 9 in, 1 out]
          }
        }
        n57 = call <vilib>:"Add State(s) to Queue__jki_lib_state_machine.vi"("State(s) in (\"\")"=w163) -> ("States Out"=w162:string)  [unwired: 14 in]
      }
      frame "UI: Front Panel State" {
        # "Argument"
        # "Set Front Panel Open or Closed\n(Usage: \"UI: Front Panel State >> Open|Close\")"
        n58 = Unbundle By Name(w171) -> ("Core.Current VI Reference"=w170:refnum<vi>)
        n59 = case shown="\"Open\", Default" w169 {
          tunnel: w173 -> [w179 w192]
          tunnel: [w181 w193] -> w172
          tunnel: w170 -> [w180 w190]
          frame "Open", Default {
            n60 = property class="VI"(reference=w180, error in=w179) -> (reference out=w177:refnum<vi>, error out=w178:errorcluster, "Front Panel.Open"=w176:bool)
            n61 = case shown="True" w176 {
              tunnel: [w184 w187] -> w181
              tunnel: w178 -> [w183 w187]
              tunnel: w177 -> [w182 _]
              frame False {
                n62 = invoke class="VI" method="FP.Open"(reference=w182, error in=w183, "Activate"=TRUE, "State"=T9."Standard") -> (error out=w184:errorcluster)  [unwired: 1 in, 4 out]
              }
              frame True {
              }
            }
          }
          frame "Close" {
            n63 = property class="VI"(reference=w190, error in=w192) -> (reference out=w189:refnum<vi>, error out=w191:errorcluster, "Front Panel.Open"=w188:bool)
            n64 = case shown="True" w188 {
              tunnel: [w194 w197] -> w193
              tunnel: w191 -> [w194 w196]
              tunnel: w189 -> [_ w195]
              frame False {
              }
              frame True {
                n65 = invoke class="VI" method="FP.Close"(reference=w195, error in=w196) -> (error out=w197:errorcluster)  [unwired: 1 in, 2 out]
              }
            }
          }
        }
        n66 = call <vilib>:"Add State(s) to Queue__jki_lib_state_machine.vi"("State(s) in (\"\")"=w175) -> ("States Out"=w174:string)  [unwired: 14 in]
      }
      frame "---------- Macro ----------" {
        # "Do not put any code in this frame.\n(It is a separator no-op. You can make a copy of this frame to create a new Macro frame)"
        n67 = call <vilib>:"Add State(s) to Queue__jki_lib_state_machine.vi"("State(s) in (\"\")"=w202) -> ("States Out"=w201:string)  [unwired: 14 in]
      }
      frame "Macro: Initialize" {
        # "Initialization Macro\n(This is called once, when the VI starts)"
        n68 = call <vilib>:"Add State(s) to Queue__jki_lib_state_machine.vi"("State(s) in Front (\"\")"="Data: Initialize\nInitialize Core Data\nUI: Initialize\nUI: Front Panel State >> Open\nMacro: LOAD\nMacro: Visualize", "State(s) in (\"\")"=w208) -> ("States Out"=w207:string)  [unwired: 13 in]
      }
      frame "Macro: Exit" {
        # "Exit Macro\n(This is called once, when the VI exits)"
        n69 = Unbundle By Name(w216) -> ("Core.Close Panel on Exit?"=w215:bool)
        n70 = Select(t="UI: Front Panel State >> Close", s=w215, f="") -> (s? t:f=w212:string)
        n71 = call <vilib>:"Add State(s) to Queue__jki_lib_state_machine.vi"("State(s) in (\"\")"=w212, "State(s) at Back (\"\")"="Data: Cleanup\nExit") -> ("States Out"=w210:string)  [unwired: 13 in]
        n72 = call <vilib>:"Add State(s) to Queue__jki_lib_state_machine.vi"("State(s) in Front (\"\")"=w210, "State(s) in (\"\")"=w219) -> ("States Out"=w218:string)  [unwired: 13 in]
      }
      frame "Macro: LOAD" {
        # "Exit Macro\n(This is called once, when the VI exits)"
        n73 = property on="GENERATE BEFORE VISUALIZING" class="Bool (strict)"(error in=w225) -> (error out=w226:errorcluster, "Value"=w227:bool)  [unwired: 1 in, 1 out]
        n74 = Select(t="GENERATE: generate data\n", s=w227, f="") -> (s? t:f=w222:string)
        n75 = Concatenate Strings(w222, "LOAD: Load that .dat data\n//LOAD: Parse Comments" ("State(s) in Front (\"\")")) -> (w220:string)
        n76 = call <vilib>:"Add State(s) to Queue__jki_lib_state_machine.vi"("State(s) in Front (\"\")"=w220, "State(s) in (\"\")"=w231) -> ("States Out"=w230:string)  [unwired: 13 in]
      }
      frame "Macro: VISUALIZE" {
        # "#TODO: move loading to a speciial case"
        # "Skip or don't skip filtering step"
        # "Exit Macro\n(This is called once, when the VI exits)"
        n77 = Select(t="VISUALIZE: Apply SG Filter", s="Filter data?", f="") -> (s? t:f=w237:string)
        n78 = call <vilib>:"Add State(s) to Queue__jki_lib_state_machine.vi"("State(s) in Front (\"\")"="VISUALIZE: Initialize Cursor Graph\nVISUALIZE: Initialize Color Tables" ("State(s) in Front (\"\")"), "State(s) in (\"\")"=w237, "State(s) at Back (\"\")"="//VISUALIZE: Cursor Things\nVISUALIZE: Graph Something\nVISUALIZE: Show Processed" ("State(s) at Back (\"\")")) -> ("States Out"=w236:string)  [unwired: 12 in]
        n79 = call <vilib>:"Add State(s) to Queue__jki_lib_state_machine.vi"("State(s) in Front (\"\")"=w236, "State(s) in (\"\")"=w243) -> ("States Out"=w242:string)  [unwired: 13 in]
      }
      frame "---------- GENERATE ----------" {
        # "Template Separator\n(You can make a copy of, or modify, this frame)"
        n80 = call <vilib>:"Add State(s) to Queue__jki_lib_state_machine.vi"("State(s) in (\"\")"=w248) -> ("States Out"=w247:string)  [unwired: 14 in]
      }
      frame "GENERATE: generate data" {
        # "Template Separator\n(You can make a copy of, or modify, this frame)"
        n81 = call "ZGenerate.vi"("File Information"="File Information", "attempt to fix filtered time?"="attempt to fix filtered time?", "decimating factor for generation"="decimating factor for generation", "offset"="offset", "length"="length", "error in"=w256, "increment (T) or overwrite (F) folders"="increment (T) or overwrite (F) folders") -> ("error out"=w249:errorcluster)  [unwired: 6 in, 2 out]
        n82 = call <vilib>:"Add State(s) to Queue__jki_lib_state_machine.vi"("State(s) in (\"\")"=w260) -> ("States Out"=w259:string)  [unwired: 14 in]
      }
      frame "---------- LOAD ----------" {
        # "Template Separator\n(You can make a copy of, or modify, this frame)"
        n83 = call <vilib>:"Add State(s) to Queue__jki_lib_state_machine.vi"("State(s) in (\"\")"=w265) -> ("States Out"=w264:string)  [unwired: 14 in]
      }
      frame "LOAD: Load that .dat data" {
        w305 = 1
        # "# itx, # chan, # samp"
        # "#TODO fix this abomination"
        # "Get root processed directory"
        # "#TODO gotta fix this when adding multiple dimensions,\nthis is actually vslow*vfast*vslowest"
        # "unflatten 1D arrays to 3D"
        n84 = property on="increment (T) or overwrite (F) folders" class="Bool (strict)"() -> ("Value"=w297:bool)  [unwired: 2 in, 2 out]
        n85 = property on="File Information" class="Clust (strict)"() -> ("Value"=w295:T6)  [unwired: 2 in, 2 out]
        n86 = control-ref of="loading"() -> (w310:refnum<vi>)
        n87 = property class="Bool (strict)"(reference=w310, error in=w272, "Value"=TRUE) -> (reference out=w311:refnum<vi>, error out=w286:errorcluster)
        n88 = flat-sequence {
          tunnel: w273 -> [w322]
          tunnel: [w322] -> w272
          tunnel: [w321] -> w271
          frame #0 {
            n89 = call "Get Windows Process Memory Usage.vi"() -> ("Memory Used By This Process (KB)"=w321:dbl)  [unwired: 11 in]
          }
        }
        n90 = call "ZDataVIS_get_processed_directory.vi"("increment (T) or overwrite (F) folders"=w297, "File Information"=w295) -> ("modified path"=w280:path)  [unwired: 9 in]
        n91 = Build Path(base path=w280, name or relative path="index.dat") -> (appended path=w288:path)
        n92 = call "DataVIS_Read Index .DAT Data.vi"("file path (use dialog)"=w288) -> ("itx # info"=w276:i32[], "channel / path dictionary"=w284:T16)  [unwired: 8 in, 1 out]
        n93 = call <userlib>:"Dictionary Get Keys__ogtk.vi"("error in (no error)"=w286, "dictionary"=w284) -> ("error out"=w285:errorcluster, "keys"=w283:variant[])  [unwired: 7 in, 1 out]
        n94 = Variant To Data(type=string[] [], Variant=w283) -> (data=w278:string[])  [unwired: 1 in, 1 out]
        n95 = flat-sequence {
          tunnel: w278 -> [w324]
          tunnel: w278 -> [w323]
          tunnel: [w325] -> w282
          tunnel: [w328] -> w281
          frame #0 {
            n96 = property on="Vsd" class="Ring (strict)"("Strings []"=w323) -> ()  [unwired: 2 in, 2 out]
            n97 = property on="I" class="Ring (strict)"("Strings []"=w324) -> ()  [unwired: 2 in, 2 out]
          }
          frame #1 {
            n98 = property on="I" class="Ring (strict)"() -> ("RingText.Text"=w326:string)  [unwired: 2 in, 2 out]
            n99 = property on="Vsd" class="Ring (strict)"() -> ("RingText.Text"=w329:string)  [unwired: 2 in, 2 out]
            n100 = Concatenate Strings(w326, ".dat") -> (w325:string)
            n101 = Concatenate Strings(w329, ".dat") -> (w328:string)
          }
        }
        n102 = Build Path(base path=w280, name or relative path="LOCKIN INFO.dat") -> (appended path=w289:path)
        n103 = Build Path(base path=w280, name or relative path=w281) -> (appended path=w293:path)
        n104 = Build Path(base path=w280, name or relative path=w282) -> (appended path=w294:path)
        n105 = call "DataVIS_Read .DAT Data.vi"("error in (no error)"=w285, "file path (use dialog)"=w294) -> ("error out"=w291:errorcluster, "all stacked channels"=w302:dbl[])  [unwired: 8 in]
        n106 = call "DataVIS_Read .DAT Data.vi"("error in (no error)"=w291, "file path (use dialog)"=w293) -> ("error out"=w290:errorcluster, "all stacked channels"=w308:dbl[])  [unwired: 8 in]
        n107 = call "DataVIS_Read Lockin .DAT Data.vi"("error in (no error)"=w290, "file path (use dialog)"=w289) -> ("error out"=w287:errorcluster, "AO DC"=w301:dbl[][])  [unwired: 6 in, 2 out]
        n108 = Index Array(array=w276) -> (element #1=w275:i32, element #3=w274:i32)  [unwired: 3 in, 1 out]
        n109 = Bundle By Name(cluster=T10 {"# Vslow"=4, "# Vfast"=10, "# Vslowest"=1, "# Samples per IV"=3130} ("sampling info"), "# Vslow"=w305, "# Vfast"=w275, "# Vslowest"=w305, "# Samples per IV"=w274) -> (w306:T10)
        n110 = Index Array(array=w301, index (row)=1) -> (element=w277:dbl[])  [unwired: 1 in]
        "Vfast" <- w277
        n111 = call "ZDataVIS_Unflatten.vi"("diff points"="Differential Bin", "sampling info"=w306, "Vsd"=w308, "I"=w302) -> ("DVR ready"=w303:T8, 4:→"mem after unflatten", 6:→"mem before unflatten")  [unwired: 3 in, 2 out]
        n112 = Build Array(w277) -> (w300:dbl[][])
        n113 = New Data Value Reference(data value=w303, error in=w287) -> (data value reference=w304:refnum<data-value>, error out=w314:errorcluster)
        n114 = Bundle By Name(cluster=w316, "Data DVR"=w304, "Sweep Data Cluster.Vfast"=w300) -> (w270:T11)
        n115 = call <vilib>:"Add State(s) to Queue__jki_lib_state_machine.vi"("State(s) in (\"\")"=w318) -> ("States Out"=w317:string)  [unwired: 14 in]
        n116 = property class="Bool (strict)"(reference=w311, error in=w314, "Value"=FALSE) -> (error out=w313:errorcluster)  [unwired: 1 out]
        n117 = flat-sequence {
          tunnel: [w320] -> w268
          tunnel: w270 -> [w319]
          tunnel: [w319] -> w269
          frame #0 {
            n118 = call "Get Windows Process Memory Usage.vi"() -> ("Memory Used By This Process (KB)"=w320:dbl)  [unwired: 11 in]
          }
        }
        "mem before load dat" <- w271
        "mem after load dat" <- w268
      }
      frame "LOAD: Load that OLD .dat data" {
        # "DVR"
        # "differentate and rebundle the IV data"
        # "separate meta-ish data and IV data"
        # "Read .dat file"
        n119 = control-ref of="loading"() -> (w333:refnum<vi>)
        n120 = property class="Bool (strict)"(reference=w333, error in=w339, "Value"=TRUE) -> (reference out=w334:refnum<vi>, error out=w338:errorcluster)
        n121 = call "DataVIS_Read OLD .DAT Data.vi"("error in (no error)"=w338) -> ("error out"=w345:errorcluster, "Array"=w355:T17)  [unwired: 9 in]
        n122 = Index Array(array=w355) -> (element=w356:T18)  [unwired: 1 in]
        n123 = Unbundle By Name(w356) -> ("IV-2T"=w346:cluster{dbl[], dbl[]}[][][], "IV"=w347:cluster{dbl[], dbl[]}[][][], "Vfast"=w352:dbl[][], "Vslow"=w351:dbl[], "Vslowest"=w350:dbl[], "Comments"=w349:string, "Scan names"=w343:string[])
        n124 = Bundle("Vfast"=w352, "Vslow"=w351, "Vslowest"=w350, "Comments"=w349, "Scan names"=w343) -> (w348:T14)  [unwired: 1 in]
        n125 = property on="Differential Bin" class="DigNum (strict)"() -> ("Value"=w331:dbl)  [unwired: 2 in, 2 out]
        n126 = call "DataVIS_Differentiate_and_Rebundle.vi"("Fit Points"=w331, "error in (no error)"=w345, "IV"=w347, "IV-2T"=w346) -> ("error out"=w344:errorcluster, "Data Cell"=w342:T8)  [unwired: 6 in]
        n127 = New Data Value Reference(data value=w342, error in=w344) -> (data value reference=w341:refnum<data-value>, error out=w337:errorcluster)
        n128 = Bundle By Name(cluster=w354, "Data DVR"=w341, "Sweep Data Cluster"=w348, "Scan names"=w343) -> (w353:T11)
        n129 = property class="Bool (strict)"(reference=w334, error in=w337, "Value"=FALSE) -> (error out=w336:errorcluster)  [unwired: 1 out]
        n130 = call <vilib>:"Add State(s) to Queue__jki_lib_state_machine.vi"("State(s) in (\"\")"=w358) -> ("States Out"=w357:string)  [unwired: 14 in]
      }
      frame "LOAD: Parse Comments" {
        n131 = Unbundle By Name(w362) -> ("Sweep Data Cluster.Comments"=w360:string)
        n132 = disable-structure shown="Disabled" {
          disable-tunnel: w360 -> [w373 _]
          disable-tunnel: [w369 _] -> w359
          frame Disabled {
            # "get rid of \"IGOR\" and end 'X' things"
            n133 = Search/Split String(string=w373, search string/char (-)="IGOR") -> (match + rest of string=w377:string)  [unwired: 1 in, 2 out]
            n134 = Search/Split String(string=w377, search string/char (-)="Display/R 'time") -> (substring before match=w375:string)  [unwired: 1 in, 2 out]
            n135 = call <userlib>:"Multi-line String to Array__ogtk.vi"("string"=w375) -> ("lines"=w374:string[])
            n136 = for {
              tunnel: w374 -> [w381] mode=indexing
              tunnel: [w379] -> w370 mode=indexing
              n137 = call <vilib>:"Trim Prefix.vi"("Prefix"="X//", "String"=w381) -> ("String"=w379:string)  [unwired: 9 in]
            }
            n138 = Array Subset(array=w370, index=1, length=49) -> (w368:string[])
            n139 = call "Fix_YAML.vi"("Array in"=w368) -> ("Array out"=w367:string[])  [unwired: 10 in]
            n140 = call "Parse Comments from CtlExp.vi"("ENTIRE Array of YAML Lines"=w367) -> ("wiring"=w369:string[][])  [unwired: 6 in, 3 out]
            "wiring" <- w369
          }
          frame Enabled {
          }
        }
        n141 = Bundle By Name(cluster=w362, "Wiring Configuration"=w359) -> (w364:T11)
        n142 = call <vilib>:"Add State(s) to Queue__jki_lib_state_machine.vi"("State(s) in (\"\")"=w366) -> ("States Out"=w365:string)  [unwired: 14 in]
      }
      frame "LOAD: Re-differentiate" {
        # "Your code here.\n(You can make a copy of, or modify, this frame)"
        n143 = control-ref of="update"() -> (w384:refnum<vi>)
        n144 = Unbundle By Name(w393) -> ("Data DVR"=w394:refnum<data-value>)
        n145 = property class="Bool (strict)"(reference=w384, error in=w388, "Value"=TRUE) -> (reference out=w383:refnum<vi>, error out=w387:errorcluster)
        n146 = in-place {
          in-place-border: w387 -> [w398]
          in-place-border: [w402] -> w386
          n147 = in-place-dvr #1(w394) -> (w401:T8)  [unwired: 1 out]
          n148 = property on="Differential Bin" class="DigNum (strict)"(error in=w398) -> (error out=w397:errorcluster, "Value"=w399:dbl)  [unwired: 1 in, 1 out]
          n149 = call "DataVIS_Differentiate_and_Rebundle_inPlace.vi"("Fit Points"=w399, "error in (no error)"=w397, "Data Cell In"=w401) -> ("error out"=w402:errorcluster, "Data Cell"=w400:T8)  [unwired: 7 in]
          n150 = in-place-dvr #1(w400) -> (w391:refnum<data-value>)  [unwired: 1 out]
        }
        n151 = property class="Bool (strict)"(reference=w383, error in=w386, "Value"=FALSE) -> (error out=w385:errorcluster)  [unwired: 1 out]
        n152 = Bundle By Name(cluster=w393, "Data DVR"=w391) -> (w392:T11)
        n153 = call <vilib>:"Add State(s) to Queue__jki_lib_state_machine.vi"("State(s) in (\"\")"=w396) -> ("States Out"=w395:string)  [unwired: 14 in]
      }
      frame "---------- VISUALIZE ----------" {
        # "Template Separator\n(You can make a copy of, or modify, this frame)"
        n154 = call <vilib>:"Add State(s) to Queue__jki_lib_state_machine.vi"("State(s) in (\"\")"=w407) -> ("States Out"=w406:string)  [unwired: 14 in]
      }
      frame "VISUALIZE: Sweep Cursor" {
        # "Shouldn't need to run 'graph something' again"
        # "Exit Macro\n(This is called once, when the VI exits)"
        n155 = control-ref of="2term Intensity"() -> (w424:refnum<vi>)
        n156 = Unbundle By Name(w432) -> ("Arr of Y arrays (intensity info)"=w431:dbl[][])
        n157 = property on="tpose" class="Bool (strict)"() -> ("Value"=w412:bool)  [unwired: 2 in, 2 out]
        n158 = Index Array(array=w431) -> (element=w430:dbl[])  [unwired: 2 in]
        n159 = Array Size(array=w431) -> (size(s)=w429:i32[])
        n160 = Index Array(array=w429) -> (element=w409:i32)  [unwired: 1 in]
        "y direction" <- w409
        n161 = Array Size(array=w430) -> (size(s)=w411:i32)
        "x direction" <- w411
        n162 = case shown="False" w412 {
          tunnel: w411 -> [w436 w437]
          tunnel: [w436 w438] -> w410
          tunnel: w409 -> [w435 w438]
          tunnel: [w435 w437] -> w408
          frame False {
          }
          frame True {
          }
        }
        n163 = case shown="\"Y\"" "x or y sweep" {
          tunnel: w408 -> [_ w448]
          tunnel: w423 -> [w443 w450]
          tunnel: w424 -> [w444 w449]
          tunnel: w410 -> [w445 _]
          tunnel: [w445 w448] -> w419
          tunnel: w416 -> [w442 w447]
          tunnel: [w441 w446] -> w415
          frame "X", Default {
            n164 = property class="IntGraph (strict)"(reference=w444, error in=w442, "Cursor.Cursor Plot"=w443) -> (error out=w441:errorcluster)  [unwired: 1 out]
          }
          frame "Y" {
            n165 = property class="IntGraph (strict)"(reference=w449, error in=w447, "Cursor.Cursor Index"=w450) -> (error out=w446:errorcluster)  [unwired: 1 out]
          }
        }
        n166 = case shown="False" "loop ctl" {
          tunnel: ["" "Event Structure\nVISUALIZE: Show Processed\nVISUALIZE: Sweep Cursor"] -> w414
          frame False {
          }
          frame True {
          }
        }
        n167 = Subtract(x=w419, y=1) -> (x-y=w420:i32)
        n168 = Less?(x=w423, y=w420) -> (x < y?=w422:bool)
        n169 = Select(t="Event Structure\nVISUALIZE: Show Processed\nVISUALIZE: Sweep Cursor", s=w422, f=w414) -> (s? t:f=w428:string)
        n170 = case shown="False" w422 {
          tunnel: w423 -> [_ w453]
          tunnel: [0 w452] -> w426
          frame False {
          }
          frame True {
            n171 = Increment(x=w453) -> (x+1=w452:i32)
          }
        }
        n172 = call <vilib>:"Add State(s) to Queue__jki_lib_state_machine.vi"("State(s) in (\"\")"=w434, "State(s) at Back (\"\")"=w428) -> ("States Out"=w433:string)  [unwired: 13 in]
        n173 = call <userlib>:"Wait (ms)__ogtk.vi"("error in (no error)"=w415, "milliseconds to wait"="ms to wait") -> ("error out"=w417:errorcluster)  [unwired: 8 in, 1 out]
      }
      frame "VISUALIZE: Show Processed" {
        # "#TODO make these subvis"
        # "update with switching"
        # "#TODO i need to look at this"
        # "Line Cuts"
        # "Template Separator\n(You can make a copy of, or modify, this frame)"
        n174 = Unbundle By Name(w469) -> ("Scan names"=w474:string[], "Decimated X values"=w475:dbl[], "X Step Info"=w463:cluster{"X Low":dbl, "X High":dbl, "X Step":dbl})  [unwired: 2 out]
        n175 = Unbundle(w463) -> ("X High"=w462:dbl)  [unwired: 2 out]
        n176 = call "ZDataVIS_XY_Offset+Mult.vi"("error in (no error)"=w472, "State Wire IN"=w469) -> ("error out"=w483:errorcluster, "Y Offset+Mult"=w461:cluster{"Offset X Low":dbl, "X Step":dbl}, "X Offset+Mult"=w464:cluster{"Offset X Low":dbl, "X Step":dbl}, "State Wire OUT"=w481:T11)  [unwired: 6 in]
        n177 = case shown="True" "-X" {
          tunnel: w464 -> [w486 w490]
          tunnel: [w486 w491] -> w456
          tunnel: w462 -> [_ w487]
          frame False {
          }
          frame True {
            n178 = Unbundle(w490) -> ("X Step"=w489:dbl)  [unwired: 1 out]
            n179 = Negate(x=w489) -> (-x=w488:dbl)
            n180 = Bundle("X High"=w487, w488) -> (w491:cluster{"X High":dbl, dbl})  [unwired: 1 in]
          }
        }
        n181 = control-ref of="2term Intensity"() -> (w455:refnum<vi>)
        n182 = property on="Y AXIS" class="LstBox (strict)"() -> ("Value"=w454:i32)  [unwired: 2 in, 2 out]
        n183 = property on="Z Axis" class="Enum (strict)"() -> ("Value"=w470:T3)  [unwired: 2 in, 2 out]
        n184 = property on="X AXIS" class="LstBox (strict)"() -> ("Value"=w466:i32)  [unwired: 2 in, 2 out]
        n185 = call "ZDataVIS_LineCuts.vi"("Intensity Plot"=w455, "e^2/h?"="e^2/h?", "tpose"=FALSE, "error in (no error)"=w483, "Decimated X values"=w475, "State Wire IN"=w481) -> ("error out"=w482:errorcluster, "X line cut"=→"Source-drain Current vs Voltage":cluster{dbl[], dbl[]}, "Y line cut"=→"Source-drain Current vs Side Gate Voltage":cluster{"Vfast":dbl[], dbl[]}, "State Wire OUT"=w468:T11)  [unwired: 2 in]
        n186 = Bundle("Value"=w466, "Value"=w454, "Value"=w470) -> (w460:T19)  [unwired: 1 in]
        n187 = property on="tpose" class="Bool (strict)"() -> ("Value"=w459:bool)  [unwired: 2 in, 2 out]
        n188 = control-ref of="Source-drain Current vs Voltage"() -> (w477:refnum<vi>)
        n189 = call "ZDataVIS_Configure_Intensity_Plot.vi"("swap x and y?"=w459, "autoName"="autoName axes", "XYZ Variable Selection"=w460, "Scan Name"=w474, "error in (no error)"=w482, "Y Offset and Multiplier"=w461, "X Offset and Multiplier"=w456, "IntensityGraph in"=w455) -> ("error out"=w473:errorcluster)  [unwired: 3 in]
        n190 = control-ref of="Source-drain Current vs Side Gate Voltage"() -> (w479:refnum<vi>)
        n191 = call <vilib>:"Add State(s) to Queue__jki_lib_state_machine.vi"("State(s) in (\"\")"=w485) -> ("States Out"=w484:string)  [unwired: 14 in]
        n192 = call "ZDataVIS_Configure_Linecuts.vi"("IntensityGraph in"=w455, "XYZ Variable Selection"=w460, "Scan Name"=w474, "error in (no error)"=w473, "swap x and y?"=w459, "Y line cut"=w479, "X line cut"=w477) -> ("error out"=w471:errorcluster)  [unwired: 4 in]
      }
      frame "VISUALIZE: Graph Something" {
        # "#TODO: if it's slow, keep the main looping INSIDE this"
        n193 = Unbundle By Name(w500) -> ("Data DVR"=w497:refnum<data-value>, "Cursor Info.Slow Index"=w496:dbl, "Cursor Info.Fast Index"=w494:dbl[])  [unwired: 2 out]
        n194 = call "Get Windows Process Memory Usage.vi"() -> ("Memory Used By This Process (KB)"=w492:dbl)  [unwired: 11 in]
        n195 = in-place {
          in-place-border: w496 -> [w529]
          in-place-border: w500 -> [w519]
          in-place-border: [w538] -> w501
          in-place-border: w502 -> [w537]
          in-place-border: [w504] -> w495
          in-place-border: w494 -> [w532]
          in-place-border: w492 -> [w506]
          # "#TODO make these subvis"
          # "Make X control\ncome from X AXIS control"
          # "light the light in case it hasn't been already"
          # "Turn off the update indicator when it is done updating"
          # "update cursor"
          # "Decimate it"
          n196 = in-place-dvr #2(w497) -> (w534:T8)  [unwired: 1 out]
          n197 = Index Array(array=w532, index=0) -> (element=w530:dbl)
          n198 = control-ref of="update"() -> (w536:refnum<vi>)
          n199 = property class="Bool (strict)"(reference=w536, error in=w537, "Value"=TRUE) -> (error out=w522:errorcluster)  [unwired: 1 out]
          n200 = Bundle("Slow Index"=w529, "Field/Temperature"="Field/Temperature", w530) -> (w528:T20)  [unwired: 1 in]
          n201 = call "ZDataVIS_SliceDataToIntensity.vi"("Y AXIS"="Y AXIS", "Z"="Z Axis", "X AXIS"="X AXIS", "error in (no error)"=w522, "Outer Indices"=w528, "Big Ol Array IN"=w534) -> ("error out"=w526:errorcluster, "Intensity Info OUT"=w527:cluster{dbl[], dbl[]}[])  [unwired: 4 in]
          n202 = call "ZDataVIS_ScaleSelect.vi"("Manual CTLs"="Manual CTLs", "Auto CTLs"="Auto CTLs", "error in (no error)"=w526, "X Scale Selection 2"="X Scale Selection", "Intensity Info IN"=w527) -> ("error out"=w542:errorcluster, "X Step Info"=w520:cluster{"X Low":dbl, "X High":dbl, "X Step":dbl}, "Intensity InfoOUT"=w509:cluster{dbl[], dbl[]}[])  [unwired: 4 in]
          n203 = call "AutoChop.vi"("use auto chop"="auto chop IV", "Intensity InfoOUT"=w509) -> ("Intensity InfoOUT 2"=w508:cluster{dbl[], dbl[]}[])  [unwired: 9 in]
          n204 = property on="-X" class="Bool (strict)"() -> ("Value"=w515:bool)  [unwired: 2 in, 2 out]
          n205 = call "ZDataVIS_Decimate+Fill_Intensity_Plot.vi"("fake point value"="Fake Point Val", "error in (no error)"=w542, "Step Info"=w520, "X and Y Arrays to decimate"=w508, "State Wire IN"=w519) -> ("error out"=w518:errorcluster, "Arr of Y arrays (intensity info)"=w514:dbl[][], "State Wire OUT"=w511:T11)  [unwired: 3 in, 1 out]
          n206 = case shown="True" w515 {
            tunnel: w514 -> [w549 w552]
            tunnel: [w549 w551] -> w513
            frame False {
            }
            frame True {
              n207 = call-poly <userlib>:"Reverse 2D Array__ogtk.vi"("by rows or columns (rows)"="-X rows or columns", "Array"=w552) -> ("Reversed Array"=w551:dbl[][])  [unwired: 1 in]
            }
          }
          n208 = case shown="True" "tpose" {
            tunnel: w513 -> [w546 w547]
            tunnel: [w546 w548] -> w517
            frame False {
            }
            frame True {
              n209 = Transpose 2D Array(2D array=w547) -> (transposed array=w548:dbl[][])
            }
          }
          n210 = case shown="True" "-Z" {
            tunnel: w517 -> [w553 w555]
            tunnel: [w553 w554] -> w510
            frame False {
            }
            frame True {
              n211 = Negate(x=w555) -> (-x=w554:dbl[][])
            }
          }
          "2term Intensity" <- w510
          n212 = Bundle By Name(cluster=w511, "Arr of Y arrays (intensity info)"=w510) -> (w505:T11)
          n213 = flat-sequence {
            tunnel: [w545] -> w504
            tunnel: w505 -> [w545]
            tunnel: [w544] -> w503
            frame #0 {
              n214 = call "Get Windows Process Memory Usage.vi"() -> ("Memory Used By This Process (KB)"=w544:dbl)  [unwired: 11 in]
            }
          }
          n215 = property class="Bool (strict)"(reference=w536, error in=w518, "Value"=FALSE ("Value (Signaling)")) -> (error out=w538:errorcluster)  [unwired: 1 out]
          n216 = in-place-dvr #2(w534) -> ()  [unwired: 2 out]
          "before 'graph something'" <- w506
          "after 'graph smoething'" <- w503
        }
        n217 = call <vilib>:"Add State(s) to Queue__jki_lib_state_machine.vi"("State(s) in (\"\")"=w499) -> ("States Out"=w498:string)  [unwired: 14 in]
      }
      frame "VISUALIZE: Apply SG Filter" {
        # "NOT IMPLEMENTED YET\n#TODO: this"
        # "Template Separator\n(You can make a copy of, or modify, this frame)"
        n218 = call <vilib>:"Add State(s) to Queue__jki_lib_state_machine.vi"("State(s) in (\"\")"=w560) -> ("States Out"=w559:string)  [unwired: 14 in]
      }
      frame "VISUALIZE: Initialize Color Tables" {
        # "#TODO:"
        # "Set color tables"
        # "Template Separator\n(You can make a copy of, or modify, this frame)"
        n219 = Reverse 1D Array(array="color scale") -> (reversed array=w564:u32[])
        n220 = call <userlib>:"Make Color Table.vi"("Array"=w564) -> ("Color Tbl"=w562:u32[])  [unwired: 1 in, 3 out]
        n221 = property on="2term Intensity" class="IntGraph (strict)"("Color Table"=w562) -> ()  [unwired: 2 in, 2 out]
        n222 = call <vilib>:"Add State(s) to Queue__jki_lib_state_machine.vi"("State(s) in (\"\")"=w568) -> ("States Out"=w567:string)  [unwired: 14 in]
      }
      frame "VISUALIZE: Initialize Cursor Graph" {
        # "scan names"
        # "Template Separator\n(You can make a copy of, or modify, this frame)"
        n223 = Unbundle By Name(w587) -> ("Sweep Data Cluster.Vfast"=w573:dbl[][], "Sweep Data Cluster.Vslow"=w575:dbl[])  [unwired: 1 out]
        n224 = Transpose 2D Array(2D array=w573) -> (transposed array=w572:dbl[][])
        n225 = Index Array(array=w572, index (col)=0 ("index (row)")) -> (element=w571:dbl[])  [unwired: 1 in]
        n226 = Index Array(array="scannn names", index #2=1 ("index")) -> (element #1=w580:string, element #2=w579:string)  [unwired: 1 in]
        n227 = for {
          tunnel: w571 -> [_] mode=indexing
          tunnel: [w596] -> _ mode=indexing
          tunnel: w575 -> [w594]
          shift-right: [w591] -> w584
          shift-left: dbl[] [] -> [w595]
          shift-right: [w593] -> w583
          shift-left: dbl[] [] -> [w592]
          tunnel: w571 -> [w590]
          n228 = Build Array (concatenate)(w595, w590) -> (w591:dbl[])
          n229 = Build Array (concatenate)(w592, w594) -> (w593:dbl[])
          n230 = Bundle(w590, "Vslow"=w594) -> (w596:cluster{dbl[], "Vslow":dbl[]})  [unwired: 1 in]
        }
        n231 = property on="Data Selection" class="XYGraph (strict)"(error in=w577, "XScale.NameLbl.Text"=w580) -> (error out=w578:errorcluster)  [unwired: 1 in, 1 out]
        n232 = property on="Data Selection" class="XYGraph (strict)"(error in=w578, "YScale.NameLbl.Text"=w579) -> (error out=w576:errorcluster)  [unwired: 1 in, 1 out]
        n233 = Bundle(w584, w583) -> (→"Data Selection":cluster{dbl[], dbl[]})  [unwired: 1 in]
        n234 = call <vilib>:"Add State(s) to Queue__jki_lib_state_machine.vi"("State(s) in (\"\")"=w589) -> ("States Out"=w588:string)  [unwired: 14 in]
      }
    }
  }
